vi "2019RefLoopPulseGen.vi"() -> ()   [LabVIEW 2017]
uses:
  offset_parameters.ctl
  Utility Sub VIs/pressure_temp_mixture.ctl
  Utility Sub VIs/pulse_generator_multiheater_controls.ctl
  Utility Sub VIs/pulse_generator_data.ctl
  Utility Sub VIs/pulse_generator_data_charts.ctl
  Utility Sub VIs/pulse_generator_data_controls.ctl
  Input Channel Lists/float_switch_physical_channels.ctl
  Input Channel Lists/pg_control_physical_channels.ctl
  Input Channel Lists/valve_physical_channels.ctl
  Input Channel Lists/window_heater_physical_channels.ctl
  Input Channel Lists/pg_motor_controller_physical_channel.ctl
  Utility Sub VIs/windows_heater_safety_values.ctl
  Utility Sub VIs/window_heaters_control.ctl
  Utility Sub VIs/power_supply_panel.ctl
  Utility Sub VIs/visual_loop.ctl
  Utility Sub VIs/diode_charts.ctl
  Utility Sub VIs/valve_pid_control.ctl
  <vilib>/Utility/error.llb/DialogType.ctl
  Input Channel Lists/label_array_cluster.ctl
  Utility Sub VIs/pulse_generator_controls_multiheater_refnums.ctl
  <vilib>/Utility/sysdir.llb/System Directory Type.ctl
  <vilib>/DAQmx/read.llb/DAQmx Read (Analog 1D Wfm NChan NSamp).vi
  <vilib>/Utility/file.llb/Write Delimited Spreadsheet (string).vi
  <vilib>/DAQmx/configure/timing.llb/DAQmx Timing (Sample Clock).vi
  <vilib>/DAQmx/miscellaneous.llb/DAQmx Fill In Error Info.vi
  <vilib>/NI Modbus.llb/MB Ethernet Master Query Read Holding Registers (poly).vi
  <vilib>/NI Modbus.llb/MB Ethernet Master Query Read Coils (poly).vi
  <vilib>/NI Modbus.llb/MB Ethernet Master Query Write Multiple Registers (poly).vi
  <vilib>/NI Modbus.llb/MB Ethernet Master Query Write Single Coil (poly).vi
  Stop_Global_Variable.vi
  <resource>/objmgr/daqmx.rc
  <vilib>/dex/Stream Element Allocation Mode.ctl
panel:
  in  "Data Saving Parameters":T1={"Sampling\nFrequency"=2000.0, "Recording Duration [s]"=1.0, "Data Index"=1, "Data Prefix"="test", "Data Folder"=path "M:/Annular Flow/Data", "Record Data"=FALSE, "Data Recording Progress"=0, "Notes: "=""} {"Data Recording Progress" scale=0.0..200000.0}
  out "notifier out":refnum<notifier>
  out "Float 5":bool
  out "Float 4":bool=TRUE
  out "Float 3":bool=TRUE
  out "Float 2":bool=TRUE
  out "Float 1":bool=TRUE
  out "Pulse Generator":u8(slide)=80 scale=0.0..100.0 scale format="%.0f%"
  out "Valve Voltage Output":dbl[](array[numeric])=[1.0, 1.0, 1.0]
  out "dataQueue":refnum<queue>
  out "autoOffsetPsatQueue":refnum<queue>
  out "start time":timestamp=timestamp(3643889234.74644 s since 1904-01-01)
  out "Seconds Since\nSession Start":dbl=73.0092568397522
  out "Time Stamp":timestamp=timestamp(3643889307.755697 s since 1904-01-01) format="%<%H:%M:%S%1u>T"
  out "Data Labels":string[][](array[string])=[["", "@(x)(12.000000*(x-0.000000)+0.000000)*6894.757290", "@(y)(y/6894.757290-0.000000)/12.000000+0.000000", "@(x)(626.174076*(x-0.004030)+0.000000)*248.840000", "@(y)(y/248.840000-0.000000)/626.174076+0.004030", "@(x)(1.000000*(x-0.000000)+0.000000)*1.000000", "@(y)(y/1.000000-0.000000)/1.000000+0.000000", "@(x)(1.000000*(x-0.000000)+0.000000)*1.000000", "@(y)(y/1.000000-0.000000)/1.000000+0.000000", "@(x)(1250.000000*(x-0.004000)+0.000000)*248.840000", "@(y)(y/248.840000-0.000000)/1250.000000+0.004000", "@(x)(156.250000*(x-0.004000)+0.000000)*6894.757290", "@(y)(y/6894.757290-0.000000)/156.250000+0.004000", "@(x)(1250.000000*(x-0.004000)+0.000000)*248.840000", "@(y)(y/248.840000-0.000000)/1250.000000+0.004000", "@(x)(1.000000*(x-0.000000)+0.000000)*1.000000", "@(y)(y/1.000000-0.000000)/1.000000+0.000000", "@(x)(1.000000*(x-0.000000)+0.000000)*1.000000", "@(y)(y/1.000000-0.000000)/1.000000+0.000000", "@(x)(10.000000*(x-0.000000)+0.000000)*6894.757290", "@(y)(y/6894.757290-0.000000)/10.000000+0.000000", "@(x)(10.000000*(x-0.000000)+0.000000)*6894.757290", "@(y)(y/6894.757290-0.000000)/10.000000+0.000000", "@(x)(0.200000*(x-0.050000)+0.000000)*6894.757290", "@(y)(y/6894.757290-0.000000)/0.200000+0.050000", "@(x)(5.000000*(x-0.000000)+0.000000)*1.000000", "@(y)(y/1.000000-0.000000)/5.000000+0.000000", "@(x)", "@(y)", "@(x)(1.000000*(x-0.000000)+0.000000)*1.000000", "@(y)(y/1.000000-0.000000)/1.000000+0.000000", "@(x)(1.000000*(x-0.000000)+0.000000)*1.000000", "@(y)(y/1.000000-0.000000)/1.000000+0.000000", "@(x)(1.000000*(x-0.000000)+0.000000)*1.000000", "@(y)(y/1.000000-0.000000)/1.000000+0.000000", "@(x)(1.000000*(x-0.000000)+0.000000)*1.000000", "@(y)(y/1.000000-0.000000)/1.000000+0.000000", "@(x)(23624.581250*(x-0.004000)+0.000000)*1.000000", "@(y)(y/1.000000-0.000000)/23624.581250+0.004000", "@(x)(125.000000*(x-0.004000)+0.000000)*1.000000", "@(y)(y/1.000000-0.000000)/125.000000+0.004000", "@(x)(23624.581250*(x-0.004000)+0.000000)*1.000000", "@(y)(y/1.000000-0.000000)/23624.581250+0.004000", "@(x)(125.000000*(x-0.004000)+0.000000)*1.000000", "@(y)(y/1.000000-0.000000)/125.000000+0.004000", "@(x)(1.000000*(x-0.000000)+0.000000)*1.000000", "@(y)(y/1.000000-0.000000)/1.000000+0.000000", "@(x)(10.000000*(x-0.000000)+0.000000)*6894.757290", "@(y)(y/6894.757290-0.000000)/10.000000+0.000000", "@(x)(1.000000*(x-0.000000)+0.000000)*1.000000", "@(y)(y/1.000000-0.000000)/1.000000+0.000000", "@(x)(10.000000*(x-0.000000)+0.000000)*6894.757290", "@(y)(y/6894.757290-0.000000)/10.000000+0.000000", "@(x)(1.000000*(x-0.000000)+0.000000)*1.000000", "@(y)(y/1.000000-0.000000)/1.000000+0.000000", "@(x)(10.000000*(x-0.000000)+0.000000)*6894.757290", "@(y)(y/6894.757290-0.000000)/10.000000+0.000000", "@(x)(1.000000*(x-0.000000)+0.000000)*1.000000", "@(y)(y/1.000000-0.000000)/1.000000+0.000000", "@(x)(12.000000*(x-0.000000)+0.000000)*6894.757290", "@(y)(y/6894.757290-0.000000)/12.000000+0.000000", "@(x)(10.000000*(x-0.000000)+0.000000)*6894.757290", "@(y)(y/6894.757290-0.000000)/10.000000+0.000000", "@(x)(6.250000*(x-1.000000)+0.000000)*6894.757290", "@(y)(y/6894.757290-0.000000)/6.250000+1.000000", "@(x)", "@(y)", "@(x)(10.000000*(x-0.000000)+0.000000)*6894.757290", "@(y)(y/6894.757290-0.000000)/10.000000+0.000000", "@(x)(1.000000*(x-0.000000)+0.000000)*1.000000", "@(y)(y/1.000000-0.000000)/1.000000+0.000000", "@(x)(10.000000*(x-0.000000)+0.000000)*6894.757290", "@(y)(y/6894.757290-0.000000)/10.000000+0.000000", "@(x)(1.000000*(x-0.000000)+0.000000)*1.000000", "@(y)(y/1.000000-0.000000)/1.000000+0.000000", "@(x)(1.000000*(x-0.000000)+0.000000)*1.000000", "@(y)(y/1.000000-0.000000)/1.000000+0.000000"], ["Timestamp", "PGAbsolutePressure Raw", "PGAbsolutePressure", "VenturidP Raw", "VenturidP", "PGVaporTemperature Raw", "PGVaporTemperature", "PGLiquidTemperature Raw", "PGLiquidTemperature", "Window1to4dP Raw", "Window1to4dP", "Window1to7FastdP Raw", "Window1to7FastdP", "Window1to7dP Raw", "Window1to7dP", "CH4 Raw", "CH4", "CH5 Raw", "CH5", "TSWindow1AbsolutePressure Raw", "TSWindow1AbsolutePressure", "TSWindow7AbsolutePressure Raw", "TSWindow7AbsolutePressure", "DwyerdP Raw", "DwyerdP", "CameraVoltage Raw", "CameraVoltage", "Power Raw", "Power", "MainDiode Raw", "MainDiode", "ControlDiode Raw", "ControlDiode", "TSExteriorTemperature Raw", "TSExteriorTemperature", "DSExteriorTemperature Raw", "DSExteriorTemperature", "VaporMassFlow Raw", "VaporMassFlow", "VaporLineDensity Raw", "VaporLineDensity", "LiquidMassFlow Raw", "LiquidMassFlow", "LiquidLineDensity Raw", "LiquidLineDensity", "MegaTankTemperature Raw", "MegaTankTemperature", "MegaTankPressure Raw", "MegaTankPressure", "SeparatorTemperature Raw", "SeparatorTemperature", "SeparatorPressure Raw", "SeparatorPressure", "LiquidInletTemperature Raw", "LiquidInletTemperature", "LiquidInletPressure Raw", "LiquidInletPressure", "UpperDevSectionTemperature Raw", "UpperDevSectionTemperature", "UpperDevSectionPressure Raw", "UpperDevSectionPressure", "LowerDevSectionPressure Raw", "LowerDevSectionPressure", "AtmosphericPressure Raw", "AtmosphericPressure", "MixingTeedP Raw", "MixingTeedP", "PGinlet-MixingTeePressure Raw", "PGinlet-MixingTeePressure", "PGinlet-MixingTeeTemperature Raw", "PGinlet-MixingTeeTemperature", "TestSectionPressure Raw", "TestSectionPressure", "CH8 Raw", "CH8", "CH9 Raw", "CH9"]]
  in  "Tab Control":T2(tab)=enum."Pulse Generator Data"
  in  "Tabulated/Visualized":enum32{"Tabulated", "Visualized"}(tab)
  in  "Zero Pressure Offsets":bool
  in  "Zero Temp Offsets":bool
  out "Pressure/Temperature/Mixture Properties":T3={"Line Densities\n[g/cm^3]"={"Vapor Line"=-0.500242358953125, "Liquid Line"=-0.5002218156718748}, "Mixture Properties"={"Enthalpy"=328364.73121574003, "Quality [-]"=0.5342547124001654}, "Component PTs"={"Liquid Tank P"=-238.37326971310944, "Liquid Tank T"=19.354366294786907, "Liquid Tank Sat P"=119198.0966686119, "Liquid Tank Sat T"=nan, "Separator P"=641.3597640511042, "Separator T"=19.076846611835087, "Separator Sat P"=117956.20227295622, "Separator Sat T"=-123.53943823013691, "Liquid Inlet P"=-411.8632841584256, "Liquid Inlet T"=19.379355794062125, "Liquid Inlet Sat P"=119310.56377459057, "Liquid Inlet Sat T"=nan, "Vapor Tank P"=-6643.862400161957, "Vapor Tank T"=19.22986162222596, "Vapor Tank Sat P"=118639.33205152737, "Vapor Tank Sat T"=nan, "Vapor Inlet P"=-6643.862400161957, "Vapor Inlet T"=19.22986162222596, "Vapor Inlet Sat P"=118639.33205152737, "Vapor Inlet Sat T"=nan, "Test Section P"=1430.2440274795968, "Test Section T"=0.0, "Test Section Sat P"=57418.5, "Test Section Sat T"=-101.60350769439742, "Upper Dev Section P"=-36.154383120368585, "Upper Dev Section T"=19.182874456914785, "Upper Dev Section Sat P"=118429.13976409887, "Upper Dev Section Sat T"=nan, "Lower Dev Section P"=893.1891396173642, "Lower Dev Section T"=19.182874456914785, "Lower Dev Section Sat P"=118429.13976409887, "Lower Dev Section Sat T"=-114.48050725695731}, "Ambient Pressure [Pa]"=-43212.87918250694, "Mixing Tee"={"Venturi dP"=0.0, "PGminiPressure"=-6216.731665575269, "PGminiTemperature"=19.20694540664635}}
  in  "Auto Offset":bool
  in  "Offset Parameters":T4
  out "Auto Offset Progress":u32(slide) scale=0.0..20.0
  out "# of Datasets Processed":i32=689
  out "Visual Loop Display":T5={"VpTkTemp"=19.22986162222596, "VpTkPres"=-6642.107688688032, "LiqTkTemp"=19.354366294786907, "LiqTkPres"=-236.9015763087729, "PGVapTemp"=18.97439824494449, "PgPres"=-41.11285782633792, "VapInTemp"=19.22986162222596, "VapInPres"=-6642.107688688032, "SepTemp"=19.076846611835087, "SepPres"=645.718240655613, "TSInTemp"=897.2079946562989, "TSInPres"=-34.66004827761057, "LiqInTemp"=19.379355794062125, "LiqInPres"=-398.1086111909236, "DevTemp"=0.0, "DevPres"=0.0, "TSTemp"=0.0, "TSPres"=-43212.631541789204, "Win1-4dP"=-1244.3220538504256, "Win1-7dP"=-1244.2479135883311, "LiqMass"=-94.5155482165204, "VpMass"=-94.52992640457187, "PGMass"=0.0, "PGLiqTemp"=18.479944435977327}
  out "Camera Voltage":dbl[](graph)=[9.625728031, 9.627001843, 9.627638749, 9.629549467, 9.630823279, 9.631778638, 9.631460185, 9.633370903, 9.633689356, 9.633689356, 9.634007809, 9.633370903, 9.633370903, 9.633689356, 9.632415544, 9.632733997, 9.632415544, 9.631778638, 9.630186373, 9.631141732, 9.629231014, 9.628275655, 9.62668339, 9.624772672, 9.62349886, 9.622543501, 9.622225048, 9.622225048, 9.622543501, 9.624135766, 9.625091125, 9.625409578000001, 9.627001843, 9.627638749, 9.629231014, 9.628594108, 9.630186373, 9.631460185, 9.632733997, 9.632733997, 9.633370903, 9.634326262, 9.634007809, 9.634644715, 9.634326262, 9.634963168, 9.635281621, 9.634644715, 9.634007809, 9.633689356, 9.633052450000001, 9.631141732, 9.631141732, 9.629231014, 9.627320296, 9.625728031, 9.624454219, 9.623180407, 9.621906595, 9.620951236, 9.620632783, 9.620951236, 9.622225048, 9.623180407, 9.62349886, 9.624454219, 9.626046484, 9.627638749, 9.628275655, 9.62986792, 9.631141732, 9.632097091, 9.633052450000001, 9.634007809, 9.634326262, 9.634644715, 9.635600074000001, 9.635281621, 9.635600074000001, 9.634963168, 9.634644715, 9.633689356, 9.633689356, 9.633052450000001, 9.632733997, 9.631460185, 9.630504826000001, 9.628912561, 9.627001843, 9.625728031, 9.62349886, 9.621906595, 9.620951236, 9.620632783, 9.620951236, 9.620314330000001, 9.621906595, 9.622861954000001, 9.624135766, 9.624772672, 9.626046484, 9.627957202000001, 9.628912561, 9.630186373, 9.631141732, 9.632097091, 9.632733997, 9.633370903, 9.634963168, 9.635281621, 9.635600074000001, 9.635918527, 9.635600074000001, 9.635918527, 9.635918527, 9.634326262, 9.634326262, 9.632733997, 9.632097091, 9.631141732, 9.62986792, 9.628275655, 9.62668339, 9.624772672, 9.622861954000001, 9.622225048, 9.621588142, 9.621588142, 9.621906595, 9.621588142, 9.622543501, 9.623180407, 9.62349886, 9.625091125, 9.62668339, 9.628594108, 9.628912561, 9.630504826000001, 9.631778638, 9.632097091, 9.633052450000001, 9.633689356, 9.634326262, 9.634644715, 9.634326262, 9.634963168, 9.635281621, 9.634963168, 9.634644715, 9.634644715, 9.634644715, 9.634007809, 9.632415544, 9.630504826000001, 9.629549467, 9.627957202000001, 9.625091125, 9.624135766, 9.622543501, 9.621269689, 9.620951236, 9.621906595, 9.622225048, 9.622543501, 9.62349886, 9.624454219, 9.625409578000001, 9.626364937, 9.627001843, 9.627320296, 9.628912561, 9.630186373, 9.631141732, 9.631778638, 9.632097091, 9.632415544, 9.633052450000001, 9.633689356, 9.634326262, 9.634326262, 9.634326262, 9.634326262, 9.633689356, 9.633052450000001, 9.632415544, 9.631778638, 9.630823279, 9.629549467, 9.628275655, 9.62668339, 9.625409578000001, 9.624135766, 9.622225048, 9.622543501, 9.621906595, 9.622225048, 9.622861954000001, 9.62349886, 9.624135766, 9.625091125]
  out "Vapor Mass Flow Rate":T6(graph)={"Flow Set Point [g/s]"=0.0, "Flow rate [g/s]"=-94.52992640457187}
  out "Liquid Mass Flow Rate":T6(graph)={"Flow Set Point [g/s]"=0.0, "Flow rate [g/s]"=-94.5155482165204}
  in  "Vapor PID Control":T7={"Flow"={"Flow rate [g/s]"=-1.9246389316910921, "Line Density [g/cm^3]"=-0.002869791468750044}, "Valve On/Off"=FALSE, "PID Mode"=FALSE, "PLC Calc Basis"=FALSE, "Flow Set Point [g/s]"=0.0, "Pump Output [%]"=0.0, "Valve Open Voltage [V]"=3.0, "Flow Setpoint Adrs"=28872, "Pump Output Adrs"=28888, "Manual Mode Request Adrs"=16499, "Manual Mode Adrs"=16509} {"Manual Mode Adrs" format="%04x"; "Manual Mode Request Adrs" format="%04x"; "Pump Output Adrs" format="%04x"; "Flow Setpoint Adrs" format="%04x"; "Pump Output [%]" format="%.2f"; "Valve Open Voltage [V]" format="%.2f"; "Flow Set Point [g/s]" format="%.2f"}
  in  "Liquid PID Control":T7={"Flow"={"Flow rate [g/s]"=-1.0242726493384742, "Line Density [g/cm^3]"=-0.004113620409999996}, "Valve On/Off"=FALSE, "PID Mode"=FALSE, "PLC Calc Basis"=FALSE, "Flow Set Point [g/s]"=0.0, "Pump Output [%]"=0.0, "Valve Open Voltage [V]"=3.0, "Flow Setpoint Adrs"=29072, "Pump Output Adrs"=29088, "Manual Mode Request Adrs"=16599, "Manual Mode Adrs"=16609} {"Manual Mode Adrs" format="%04x"; "Manual Mode Request Adrs" format="%04x"; "Pump Output Adrs" format="%04x"; "Flow Setpoint Adrs" format="%04x"; "Pump Output [%]" format="%.2f"; "Valve Open Voltage [V]" format="%.2f"; "Flow Set Point [g/s]" format="%.2f"}
  in  "Pulse Generator Offsets":T8
  out "Measurements Data":T9={"PG Abs Pressure"=-40.9090848933398, "Vapor Temperature"=18.97439824494449, "Liquid Temperature"=18.479944435977327, "PG Supply Temperature"=-40.9090848933398, "Tinlet"=19.436676396501205, "Tsectwo"=19.49953546420568, "TS Abs Pressure W1"=-1394.614861114431, "TS Abs Pressure W7"=-1377.577180233669, "W1-4 dP[Pa]"=-1244.1716334686469, "W1-7 dP[Pa]"=-1244.2994051226024, "W1-7 dP[Pa] Fast"=-4312.785111999902, "PG Venturi dP [Pa]"=-627.9412171524315, "Vapor Line Pitot dP [Pa]"=-161.6047258814074, "Tsecthree"=19.191961040039615, "Toutlet"=19.148186089917207, "TS Ext"=18.97439824494449, "Vapor Sat Pressure"=117501.0252097072, "Liquid Sat Pressure"=115328.74681540662, "PG Mass Flow Rate"=0.0, "Vapor Line Mass Flow"=0.0}
  out "Pulse Generator Charts":T10={"Vapor Mass Flow Rates"={"max value"=0.0, "max value"=0.0}, "Test Section Thermocouples"={"[0]"=19.436676396501205, "[1]"=19.49953546420568, "[2]"=18.939848584535856, "[3]"=19.191961040039615, "[4]"=19.148186089917207}, "Pulse Generator Abs Pressure"=[-40.9090848933398], "Test Section Saturation Pressures"={"max value"=119568.94045291988, "max value"=119852.92544400034}}
  out "Diode Charts":T11={"Liquid Diodes"={10.35690505599997, 10.45756001099999}, "Liquid Intensity Ratio"=0.9903749101229978, "Vapor Diode"={0.0, 0.0}, "Vapor Intensity Ratio"=0.0, "TS Window 1 Temperatures"={"Average"=18.939848584535856, "T Sat [C]"=nan}}
  in  "Commit Settings":bool
  in  "Settings Subpanel":T12(tab)
  in  "Input":T14={"Float Switch Physical Channels"={"Float Line 1"="Input/port0/line0", "Float Line 2"="Input/port0/line1", "Float Line 3"="Input/port0/line2", "Float Line 4"="Input/port0/line3", "Float Line 5"="Input/port0/line4"}, "Float Switch Line Mode"=TRUE}
  in  "Output":T19={"Pulse Generator Control Physical Channels"={"1000W 1"="Output/port0/line1", "1000W 2"="Output/port0/line2", "1000W 3"="Output/port0/line3", "500W 1"="Output/port0/line4", "250W 1"="Output/port0/line5", "150W 1"="Output/port0/line6", "Counter Line"="cDAQ1Mod1/ctr0", "Direction Line"="cDAQ1Mod1/port0/line2"}, "Proportional Valve Physical Channels"={"Vapor Valve"="cDAQ1Mod3/ao1", "Liquid Valve"="cDAQ1Mod3/ao2"}, "Window Heaters Physical Channels"={"Front PS"="COM8", "Rear PS"="COM5"}, "Diode Communication"={"URL"="", "Serial"=""}, "PLC Communication"={"Remote IP"="192.168.0.10", "Remote Port"=502}, "PG Motor Controller Physical Channels"={"USB controller"="COM11"}}
  in  "Safety":T21={"Pulse Generator Heater Safety Values"={"Absolute Pulse Generator Pressure Limit"=250000.0, "Seconds Allowed Pulse Generator Excess Pressure"=60.0, "Absolute Pulse Generator Temperature Limit"=35.0}, "Window Heater Safety Values"={"Minimum Test Section Mass Flow "=1.0, "Maximum Test Section Temperature"=60.0}}
  in  "Import offsets":bool
  in  "Export offsets":bool
  in  "Generate MATLAB Parsing Script":bool
  in  "Open Brians VI":bool
  out "Buffer Overflow":bool
  in  "Run Log":T22(array[cluster])
  out "System Running":bool
  out "error out":errorcluster
  out "Loop Time [ms]":u32=96
  in  "Stop":bool
  in  "Tab Control 2":T23(tab)
  in  "Pulse Generator Controls":T24={"Start Pulse"=FALSE, "Stop Pulse"=FALSE, "Pulse Gen\nActive?"=FALSE, "Steady Frequency [Hz]"=10.0, "Ramp Duration [s]"=5.0, "Steady Duration[s]"=10.0, " Motor Dir"=FALSE, "Heaters"=FALSE, "Heater ON?"=FALSE, "1000-1"=FALSE, "1000-2"=FALSE, "1000-3"=FALSE, "500-1"=FALSE, "250-1"=FALSE, "150-1"=FALSE, "Hysteresis"=10.0, "PG Controller Switch"=FALSE, "Power [W]"=0.0, "Start Frequency [Hz]"=1.0, "Pulse Mode"=FALSE, "Frequency [Hz]"=0.0, "+/- % Movement"=90.0, "Repetitions"=20, "Average % Open"=90.0, "1000W 1 PID"=FALSE, "1000W 2 PID"=FALSE, "1000W 3 PID"=FALSE, "500W 1 PID"=FALSE, "250W 1 PID"=FALSE, "150W 1 PID"=FALSE, "Setpoint [Pa]"=130000.0} {"Setpoint [Pa]" min=1.0 max=5.0; "Average % Open" min=1.0 step=500.0; "+/- % Movement" min=1.0 step=500.0; "Start Frequency [Hz]" min=1.0 step=500.0; "Power [W]" min=1.0 max=5.0 format="%.2f"; "Hysteresis" min=0.0 max=5.0; "Steady Frequency [Hz]" min=1.0 step=500.0}
  in  "Window Heaters Control":T25={"Window Heater Switch"=FALSE, "Safety Trigger"=FALSE, "Front Readout"={"Voltage High Limit"=10.0, "Current High Limit"=10.0, "Power Setpoint"=2.0, "Voltage"=10.005, "Current"=0.0, "Power"=0.0}, "Rear Readout"={"Voltage High Limit"=10.0, "Current High Limit"=10.0, "Power Setpoint"=2.0, "Voltage"=9.99, "Current"=0.0007, "Power"=0.0}, "Reset PS Error"=FALSE}
  in  "Offsets":T27(array[cluster])=[{"Channel"="VaporMassFlow", "Offset"=0.0, "Output Unit"=enum."g/s"}, {"Channel"="VaporLineDensity", "Offset"=0.0, "Output Unit"=enum."g/cm3"}, {"Channel"="LiquidMassFlow", "Offset"=0.0, "Output Unit"=enum."g/s"}, {"Channel"="LiquidLineDensity", "Offset"=0.0, "Output Unit"=enum."g/cm3"}, {"Channel"="VaporInletPressure", "Offset"=0.0, "Output Unit"=enum."Pa"}, {"Channel"="MegaTankPressure", "Offset"=0.0, "Output Unit"=enum."Pa"}, {"Channel"="SeparatorPressure", "Offset"=0.0, "Output Unit"=enum."Pa"}, {"Channel"="LiquidInletPressure", "Offset"=0.0, "Output Unit"=enum."Pa"}, {"Channel"="VaporInletTemperature", "Offset"=0.0, "Output Unit"=enum."C"}, {"Channel"="MegaTankTemperature", "Offset"=0.0, "Output Unit"=enum."C"}, {"Channel"="LiquidInletTemperature", "Offset"=0.0, "Output Unit"=enum."C"}, {"Channel"="SeparatorTemperature", "Offset"=0.0, "Output Unit"=enum."C"}, {"Channel"="LowerDevSectionPressure", "Offset"=0.0, "Output Unit"=enum."Pa"}, {"Channel"="UpperDevSectionTemperature", "Offset"=0.0, "Output Unit"=enum."C"}, {"Channel"="UpperDevSectionPressure", "Offset"=0.0, "Output Unit"=enum."Pa"}, {"Channel"="TestSectionTemperature", "Offset"=0.0, "Output Unit"=enum."C"}, {"Channel"="TestSectionPressure", "Offset"=0.0, "Output Unit"=enum."Pa"}, {"Channel"="DwyerdP", "Offset"=0.0, "Output Unit"=enum."Pa"}, {"Channel"="VenturidP", "Offset"=0.0, "Output Unit"=enum."Pa"}, {"Channel"="PGinlet-MixingTeePressure", "Offset"=0.0, "Output Unit"=enum."Pa"}, {"Channel"="PGinlet-MixingTeeTemperature", "Offset"=0.0, "Output Unit"=enum."C"}, {"Channel"="AtmosphericPressure", "Offset"=0.0, "Output Unit"=enum."Pa"}, {"Channel"="PGAbsolutePressure", "Offset"=0.0, "Output Unit"=enum."Pa"}, {"Channel"="PGVaporTemperature", "Offset"=0.0, "Output Unit"=enum."C"}, {"Channel"="PGLiquidTemperature", "Offset"=0.0, "Output Unit"=enum."C"}, {"Channel"="Window1to4dP", "Offset"=0.0, "Output Unit"=enum."Pa"}, {"Channel"="Window1to7dP", "Offset"=0.0, "Output Unit"=enum."Pa"}, {"Channel"="Window1to7FastdP", "Offset"=0.0, "Output Unit"=enum."Pa"}, {"Channel"="CameraVoltage", "Offset"=0.0, "Output Unit"=enum."Volt"}, {"Channel"="CH4", "Offset"=0.0, "Output Unit"=enum."C"}, {"Channel"="CH5", "Offset"=0.0, "Output Unit"=enum."C"}, {"Channel"="TSWindow1AbsolutePressure", "Offset"=0.0, "Output Unit"=enum."Pa"}, {"Channel"="TSWindow7AbsolutePressure", "Offset"=0.0, "Output Unit"=enum."Pa"}, {"Channel"="MainDiode", "Offset"=0.0, "Output Unit"=enum."Volt"}, {"Channel"="ControlDiode", "Offset"=0.0, "Output Unit"=enum."Volt"}, {"Channel"="TSExteriorTemperature", "Offset"=0.0, "Output Unit"=enum."C"}, {"Channel"="DSExteriorTemperature", "Offset"=0.0, "Output Unit"=enum."C"}, {"Channel"="PostMixingTeeTemperature", "Offset"=0.0, "Output Unit"=enum."Volt"}, {"Channel"="CH8", "Offset"=0.0, "Output Unit"=enum."C"}, {"Channel"="CH9", "Offset"=0.0, "Output Unit"=enum."C"}]
  # "Saturation\nPressure [Pa]"
  # "Saturation\nTemperature [C]"
  # "Pressure [Pa]"
  # "Temperature [C]"
  # "Mega Tank"
  # "Separator"
  # "Liquid Inlet"
  # "Vapor Inlet"
  # "Vapor Inlet"
  # "Test Section"
  # "Upper Dev Section"
  # "Lower Dev Section"
  # "Test Section"
  # "Pulse Gen"
  # "Normal: NC\nInvert: NO\nSwitch 0 is inverted"
  # "NI-9401 Counter & DIO (pin) Chart"
  # "Default Pins used by Counter:\n     SRC: P-Gen Counter Timebase, A-input  \n     GATE: P-Gen Trigger, Z-input\n     AUX: B-input \n     OUT: P_Gen Output\nMore info:  Programs»National Instruments»NI-DAQ»NI-DAQmx Key Concepts»Counters"
  # "0"
  # "1"
  # "2"
  # "3"
  # "7 (25)"
  # "6 (23)"
  # "4 (20)"
  # "5 (22)"
  # "3 (19)"
  # "2 (17)"
  # "0 (14)"
  # "1 (16)"
  # "4 (20)"
  # "5 (22)"
  # "6 (23)"
  # "7 (25)"
  # "0 (14)"
  # "1 (16)"
  # "2 (17)"
  # "3 (19)"
  # "COUNTER"
  # "SRC"
  # "GATE"
  # "AUX"
  # "OUT"
  # "Heater Switches"
  # "Heater P Control"
  # "Current Est Power"
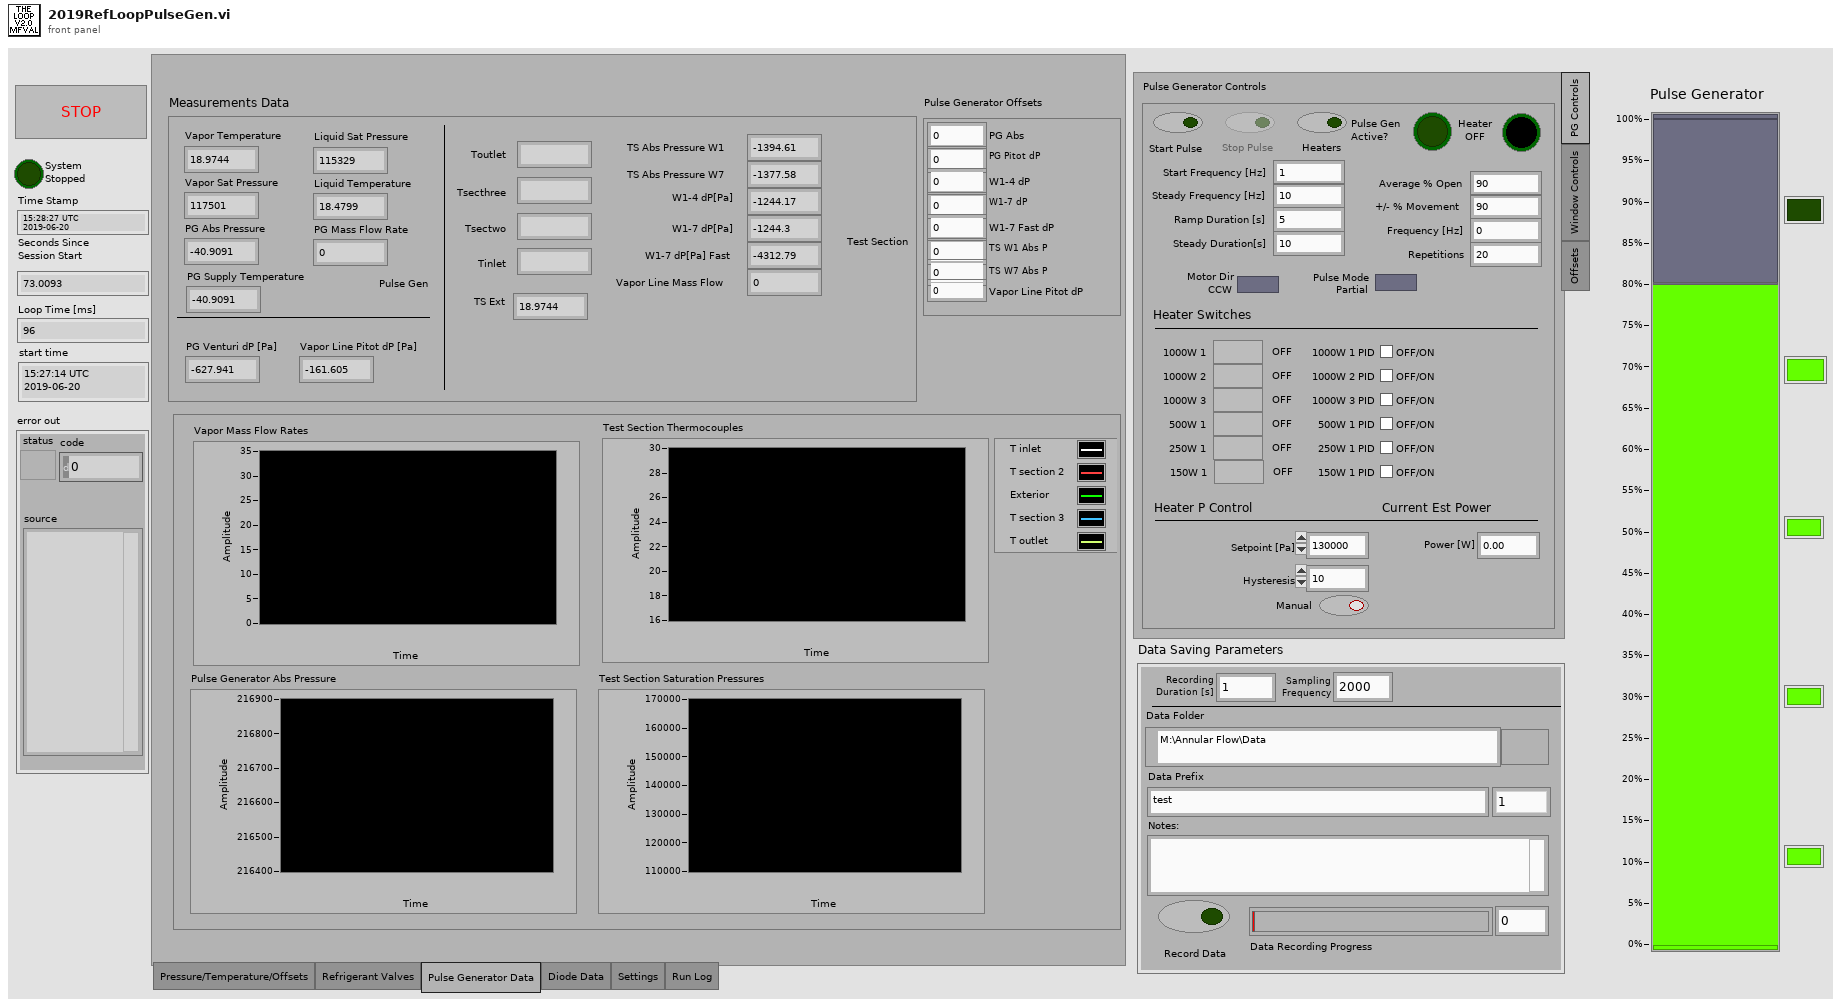
[diagram p1: front panel]
types:
  T1 = cluster{"Sampling\nFrequency":dbl, "Recording Duration [s]":dbl, "Data Index":i32, "Data Prefix":string, "Data Folder":path, "Record Data":bool, "Data Recording Progress":u32, "Notes: ":string}
  T2 = enum32{"Pressure/Temperature/Offsets", "Refrigerant Valves", "Pulse Generator Data", "Diode Data", "Settings", "Run Log"}
  T3 = typedef "pressure_temp_mixture.ctl" = cluster{"Line Densities\n[g/cm^3]":cluster{"Vapor Line":dbl, "Liquid Line":dbl}, "Mixture Properties":cluster{"Enthalpy":dbl, "Quality [-]":dbl}, "Component PTs":cluster{"Liquid Tank P":dbl, "Liquid Tank T":dbl, "Liquid Tank Sat P":dbl, "Liquid Tank Sat T":dbl, "Separator P":dbl, "Separator T":dbl, "Separator Sat P":dbl, "Separator Sat T":dbl, "Liquid Inlet P":dbl, "Liquid Inlet T":dbl, "Liquid Inlet Sat P":dbl, "Liquid Inlet Sat T":dbl, "Vapor Tank P":dbl, "Vapor Tank T":dbl, "Vapor Tank Sat P":dbl, "Vapor Tank Sat T":dbl, "Vapor Inlet P":dbl, "Vapor Inlet T":dbl, "Vapor Inlet Sat P":dbl, "Vapor Inlet Sat T":dbl, "Test Section P":dbl, "Test Section T":dbl, "Test Section Sat P":dbl, "Test Section Sat T":dbl, "Upper Dev Section P":dbl, "Upper Dev Section T":dbl, "Upper Dev Section Sat P":dbl, "Upper Dev Section Sat T":dbl, "Lower Dev Section P":dbl, "Lower Dev Section T":dbl, "Lower Dev Section Sat P":dbl, "Lower Dev Section Sat T":dbl}, "Ambient Pressure [Pa]":dbl, "Mixing Tee":cluster{"Venturi dP":dbl, "PGminiPressure":dbl, "PGminiTemperature":dbl}}
  T4 = typedef "offset_parameters.ctl" = cluster{"Mega Tank\nPressure":dbl, "Mega Tank\nTemperature":dbl, "Separator Pressure":dbl, "Separator \nTemperature":dbl, "Liquid Inlet\nPressure":dbl, "Liquid Inlet\nTemperature ":dbl, "Vapor Inlet\nPressure ":dbl, "Vapor Inlet\nTemperature ":dbl, "Vapor Inlet\nPressure":dbl, "Vapor Inlet \nTemperature":dbl, "Test Section\nPressure":dbl, "Test Section\nTemperature":dbl, "Upper Dev Section\nPressure":dbl, "Upper Dev Section\nTemperature":dbl, "Lower Dev Section\nPressure":dbl, "PG Inlet-Mixing Tee Pressure":dbl, "Vapor Line dP":dbl, "Atmospheric Pressure [Pa]":dbl}
  T5 = typedef "visual_loop.ctl" = cluster{"VpTkTemp":dbl, "VpTkPres":dbl, "LiqTkTemp":dbl, "LiqTkPres":dbl, "PGVapTemp":dbl, "PgPres":dbl, "VapInTemp":dbl, "VapInPres":dbl, "SepTemp":dbl, "SepPres":dbl, "TSInTemp":dbl, "TSInPres":dbl, "LiqInTemp":dbl, "LiqInPres":dbl, "DevTemp":dbl, "DevPres":dbl, "TSTemp":dbl, "TSPres":dbl, "Win1-4dP":dbl, "Win1-7dP":dbl, "LiqMass":dbl, "VpMass":dbl, "PGMass":dbl, "PGLiqTemp":dbl}
  T6 = cluster{"Flow Set Point [g/s]":dbl, "Flow rate [g/s]":dbl}
  T7 = typedef "valve_pid_control.ctl" = cluster{"Flow":cluster{"Flow rate [g/s]":dbl, "Line Density [g/cm^3]":dbl}, "Valve On/Off":bool, "PID Mode":bool, "PLC Calc Basis":bool, "Flow Set Point [g/s]":dbl, "Pump Output [%]":dbl, "Valve Open Voltage [V]":dbl, "Flow Setpoint Adrs":u16, "Pump Output Adrs":u16, "Manual Mode Request Adrs":u16, "Manual Mode Adrs":u16}
  T8 = typedef "pulse_generator_data_controls.ctl" = cluster{"PG Abs":dbl, "PG Pitot dP":dbl, "W1-4 dP ":dbl, "W1-7 dP":dbl, "W1-7 Fast dP":dbl, "TS W1 Abs P":dbl, "TS W7 Abs P":dbl, "Vapor Line Pitot dP":dbl}
  T9 = typedef "pulse_generator_data.ctl" = cluster{"PG Abs Pressure":dbl, "Vapor Temperature":dbl, "Liquid Temperature":dbl, "PG Supply Temperature":dbl, "Tinlet":dbl, "Tsectwo":dbl, "TS Abs Pressure W1":dbl, "TS Abs Pressure W7":dbl, "W1-4 dP[Pa]":dbl, "W1-7 dP[Pa]":dbl, "W1-7 dP[Pa] Fast":dbl, "PG Venturi dP [Pa]":dbl, "Vapor Line Pitot dP [Pa]":dbl, "Tsecthree":dbl, "Toutlet":dbl, "TS Ext":dbl, "Vapor Sat Pressure":dbl, "Liquid Sat Pressure":dbl, "PG Mass Flow Rate":dbl, "Vapor Line Mass Flow":dbl}
  T10 = typedef "pulse_generator_data_charts.ctl" = cluster{"Vapor Mass Flow Rates":cluster{"max value":dbl, "max value":dbl}, "Test Section Thermocouples":cluster{"[0]":dbl, "[1]":dbl, "[2]":dbl, "[3]":dbl, "[4]":dbl}, "Pulse Generator Abs Pressure":dbl[], "Test Section Saturation Pressures":cluster{"max value":dbl, "max value":dbl}}
  T11 = typedef "diode_charts.ctl" = cluster{"Liquid Diodes":cluster{dbl, dbl}, "Liquid Intensity Ratio":dbl, "Vapor Diode":cluster{dbl, dbl}, "Vapor Intensity Ratio":dbl, "TS Window 1 Temperatures":cluster{"Average":dbl, "T Sat [C]":dbl}}
  T12 = enum32{"Input", "Output", "Safety", "Other Functions"}
  T13 = typedef "float_switch_physical_channels.ctl" = cluster{"Float Line 1":tag, "Float Line 2":tag, "Float Line 3":tag, "Float Line 4":tag, "Float Line 5":tag}
  T14 = cluster{"Float Switch Physical Channels":T13, "Float Switch Line Mode":bool}
  T15 = typedef "pg_control_physical_channels.ctl" = cluster{"1000W 1":tag, "1000W 2":tag, "1000W 3":tag, "500W 1":tag, "250W 1":tag, "150W 1":tag, "Counter Line":tag, "Direction Line":tag}
  T16 = typedef "valve_physical_channels.ctl" = cluster{"Vapor Valve":tag, "Liquid Valve":tag}
  T17 = typedef "window_heater_physical_channels.ctl" = cluster{"Front PS":refnum<visa-resource-name>, "Rear PS":refnum<visa-resource-name>}
  T18 = typedef "pg_motor_controller_physical_channel.ctl" = cluster{"USB controller":refnum<visa-resource-name>}
  T19 = cluster{"Pulse Generator Control Physical Channels":T15, "Proportional Valve Physical Channels":T16, "Window Heaters Physical Channels":T17, "Diode Communication":cluster{"URL":string, "Serial":refnum<visa-resource-name>}, "PLC Communication":cluster{"Remote IP":string, "Remote Port":u16}, "PG Motor Controller Physical Channels":T18}
  T20 = typedef "windows_heater_safety_values.ctl" = cluster{"Minimum Test Section Mass Flow ":dbl, "Maximum Test Section Temperature":dbl}
  T21 = cluster{"Pulse Generator Heater Safety Values":cluster{"Absolute Pulse Generator Pressure Limit":dbl, "Seconds Allowed Pulse Generator Excess Pressure":dbl, "Absolute Pulse Generator Temperature Limit":dbl}, "Window Heater Safety Values":T20}
  T22 = cluster{"File Number":string, "Entry Content":string}[]
  T23 = enum32{"PG Controls", "Window Controls", "Offsets"}
  T24 = typedef "pulse_generator_multiheater_controls.ctl" = cluster{"Start Pulse":bool, "Stop Pulse":bool, "Pulse Gen\nActive?":bool, "Steady Frequency [Hz]":dbl, "Ramp Duration [s]":dbl, "Steady Duration[s]":dbl, " Motor Dir":bool, "Heaters":bool, "Heater ON?":bool, "1000-1":bool, "1000-2":bool, "1000-3":bool, "500-1":bool, "250-1":bool, "150-1":bool, "Hysteresis":dbl, "PG Controller Switch":bool, "Power [W]":dbl, "Start Frequency [Hz]":dbl, "Pulse Mode":bool, "Frequency [Hz]":dbl, "+/- % Movement":dbl, "Repetitions":u32, "Average % Open":dbl, "1000W 1 PID":bool, "1000W 2 PID":bool, "1000W 3 PID":bool, "500W 1 PID":bool, "250W 1 PID":bool, "150W 1 PID":bool, "Setpoint [Pa]":dbl}
  T25 = typedef "window_heaters_control.ctl" = cluster{"Window Heater Switch":bool, "Safety Trigger":bool, "Front Readout":T26, "Rear Readout":T26, "Reset PS Error":bool}
  T26 = typedef "power_supply_panel.ctl" = cluster{"Voltage High Limit":dbl, "Current High Limit":dbl, "Power Setpoint":dbl, "Voltage":dbl, "Current":dbl, "Power":dbl}
  T27 = cluster{"Channel":string, "Offset":dbl, "Output Unit":enum16{"psi", "Pa", "inH2O", "inHg", "C", "K", "g/s", "g/cm3", "Volt", "Amp", ""}}[]
  T28 = enum32{"Pressure/Temperature/Offsets", "Refrigerant Valves", "Pulse Generator Data", "Diode Data", "Settings"}
  T29 = enum8{"Enabled", "Disabled", "Disabled and Grayed Out"}
  T30 = cluster{"max value":dbl, "max value":dbl, "max value":dbl, "max value 2":dbl, "max value 3":dbl}[]
  T31 = enum32{"Pressure/Temperature/Offsets", "Refrigerant Valves", "Pulse Generator Data", "Settings"}
  T32 = cluster{"Channel Name":string, "Label":string, "Offset":dbl, "Raw":dbl[], "Processed":dbl[], "Converted":dbl[], "Average":dbl}
  T33 = typedef "label_array_cluster.ctl" = cluster{"Label Array":string[]}
  T34 = enum32{"Invalid", "Standard", "Closed", "Hidden", "Minimized", "Maximized"}
  T35 = cluster{"Entry Content":string, "File Number":string}
  T36 = typedef "DialogType.ctl" = u16
  T37 = cluster{"Flow Set Point [g/s]":dbl, "Flow rate [g/s]":dbl}[]
  T38 = typedef "analog_data_channel_pkg.ctl" = cluster{"Analog Input Channel":T39, "Analog Data":T40}
  T39 = typedef "input_channel.ctl" = cluster{"Channel Name":string, "Physical Channel":tag, "Sensor Type":enum16{"Absolute Pressure", "Gauge Pressure", "Differential Pressure", "Temperature", "Mass Flow Rate", "Density", "Other"}, "Signal Type":enum16{"Voltage", "Current", "Temperature"}, "Terminal Configuration":i32, "Minimum Value":dbl, "Maximum Value":dbl, "TC Type":i32, "Sensor Min":dbl, "Sensor Max":dbl, "Sensor Offset":dbl, "Sensor Unit":enum16{"psi", "Pa", "inH2O", "inHg", "C", "K", "g/s", "g/cm3", "Volt", "Amp", ""}, "Output Unit":enum16{"psi", "Pa", "inH2O", "inHg", "C", "K", "g/s", "g/cm3", "Volt", "Amp", ""}, "Unit Conversion":dbl, "Active":bool, "Input Type":enum16{"DAQ", "Add-On"}}
  T40 = typedef "analog_data.ctl" = cluster{"Label":string, "Offset":dbl, "Raw":dbl[], "Converted":dbl[], "Average":dbl, "Formula To Output":string, "Formula From Output":string}
  T41 = enum16{"psi", "Pa", "inH2O", "inHg", "C", "K", "g/s", "g/cm3", "Volt", "Amp", ""}
  T42 = cluster{"Label":string, "Offset":dbl, "Output Unit":enum16{"psi", "Pa", "inH2O", "inHg", "C", "K", "g/s", "g/cm3", "Volt", "Amp", ""}}
  T43 = typedef "index_array_cluster.ctl" = cluster{"Index Array":i32[]}
  T44 = typedef "Stream Element Allocation Mode.ctl" = u32
  T45 = cluster{"Flow":cluster{"Flow rate [g/s]":dbl, "Line Density [g/cm^3]":dbl}, "Valve On/Off":bool, "PID Mode":bool, "PLC Calc Basis":bool, "Flow Set Point [g/s]":dbl, "Pump Output [%]":dbl, "Valve Open Voltage [V]":dbl, "Flow Setpoint Adrs":u16, "Pump Output Adrs":u16, "Manual Mode Request Adrs":u16, "Manual Mode Adrs":u16}
  T46 = cluster{"Channel":string, "Offset":dbl, "Output Unit":enum16{"psi", "Pa", "inH2O", "inHg", "C", "K", "g/s", "g/cm3", "Volt", "Amp", ""}}
  T47 = typedef "pulse_generator_controls_multiheater_refnums.ctl" = cluster{"Start Pulse":refnum<vi>, "Stop Pulse":refnum<vi>, "Heaters":refnum<vi>, "Counter":refnum<vi>, "Start Frequency (Hz)":refnum<vi>, "Pulse Generator Active":refnum<vi>, "Stepper Motor Direction":refnum<vi>, "Ramp Duration":refnum<vi>, "Direction Line":refnum<vi>, "1000-1 Line":refnum<vi>, "1000-2 Line":refnum<vi>, "1000-3 Line":refnum<vi>, "500-1 Line":refnum<vi>, "250-1 Line":refnum<vi>, "1000-1":refnum<vi>, "1000-2":refnum<vi>, "1000-3":refnum<vi>, "500-1":refnum<vi>, "250-1":refnum<vi>, "150-1":refnum<vi>, "Heater ON?":refnum<vi>, "150-1 Line":refnum<vi>, "Power":refnum<vi>, "Steady Frequency (Hz)":refnum<vi>, "Steady Duration ":refnum<vi>, "Pulse Mode":refnum<vi>, "Frequency [Hz]":refnum<vi>, "Avg % Open":refnum<vi>, "Repetitions":refnum<vi>, "+/- % Open":refnum<vi>, "USB Controller":refnum<vi>}
  T48 = cluster{"Liquid Tank P":dbl, "Liquid Tank T":dbl, "Liquid Tank Sat P":dbl, "Liquid Tank Sat T":dbl, "Separator P":dbl, "Separator T":dbl, "Separator Sat P":dbl, "Separator Sat T":dbl, "Liquid Inlet P":dbl, "Liquid Inlet T":dbl, "Liquid Inlet Sat P":dbl, "Liquid Inlet Sat T":dbl, "Vapor Tank P":dbl, "Vapor Tank T":dbl, "Vapor Tank Sat P":dbl, "Vapor Tank Sat T":dbl, "Vapor Inlet P":dbl, "Vapor Inlet T":dbl, "Vapor Inlet Sat P":dbl, "Vapor Inlet Sat T":dbl, "Test Section P":dbl, "Test Section T":dbl, "Test Section Sat P":dbl, "Test Section Sat T":dbl, "Upper Dev Section P":dbl, "Upper Dev Section T":dbl, "Upper Dev Section Sat P":dbl, "Upper Dev Section Sat T":dbl, "Lower Dev Section P":dbl, "Lower Dev Section T":dbl, "Lower Dev Section Sat P":dbl, "Lower Dev Section Sat T":dbl}
  T49 = typedef "System Directory Type.ctl" = i32
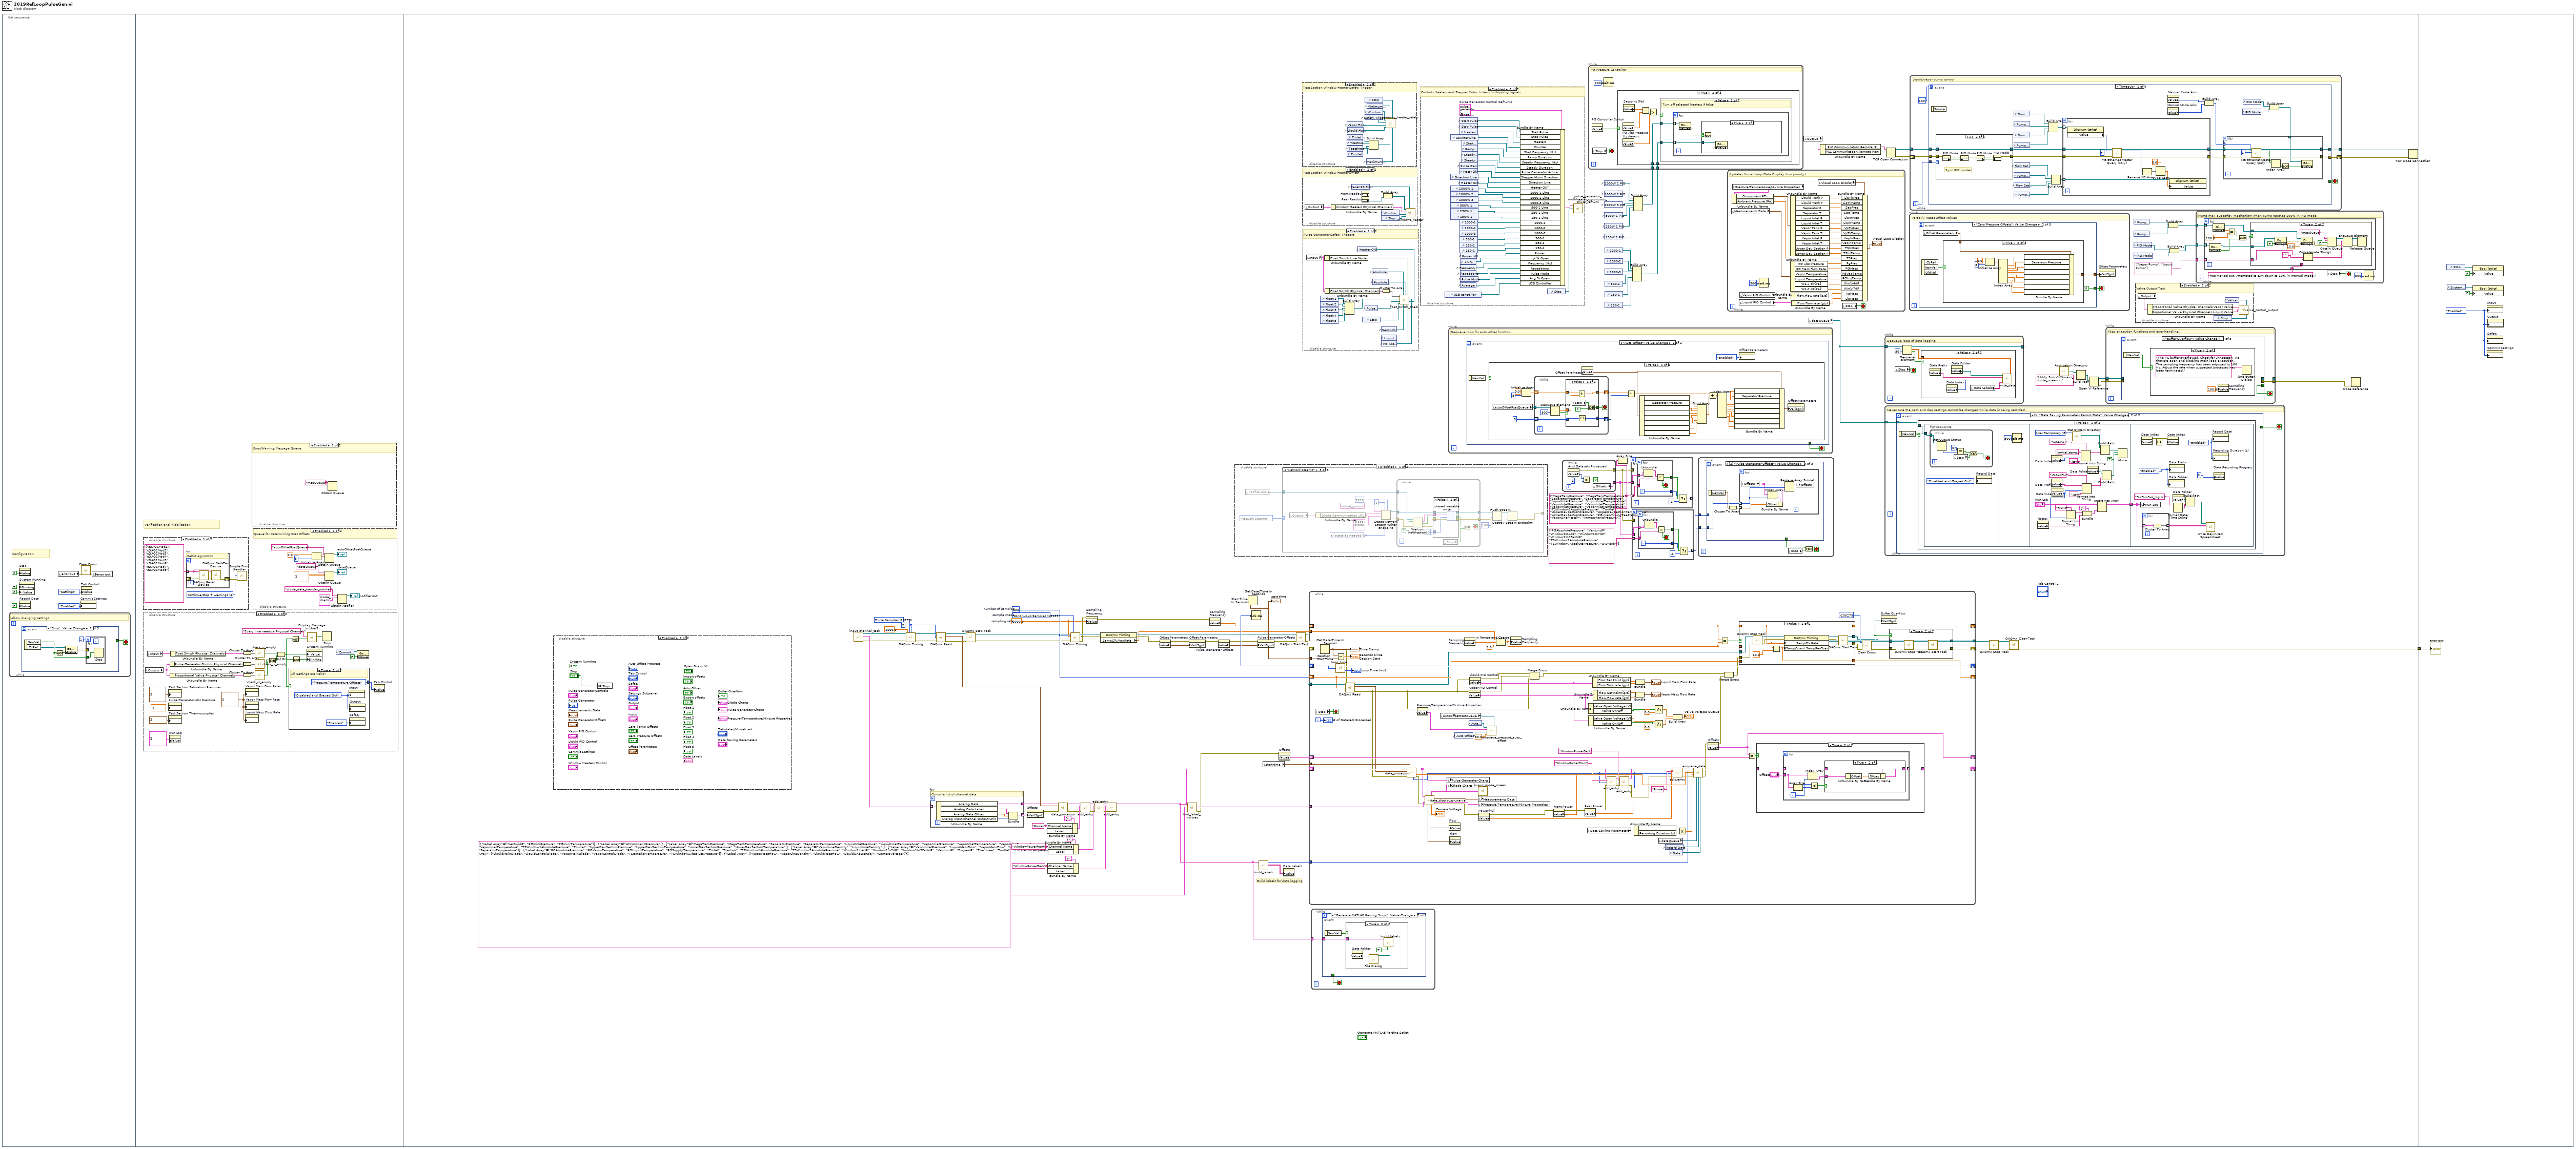
[diagram p0: block diagram]
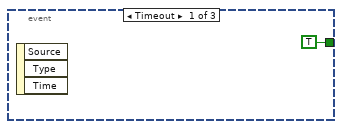
[diagram p2: hidden frame]
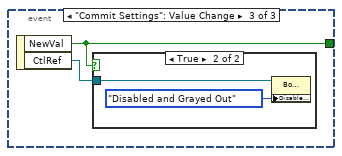
[diagram p3: hidden frame]
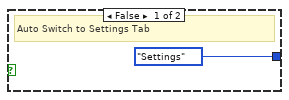
[diagram p7: hidden frame]
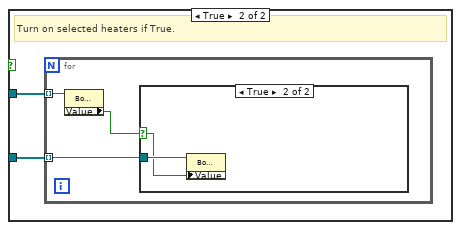
[diagram p13: hidden frame]
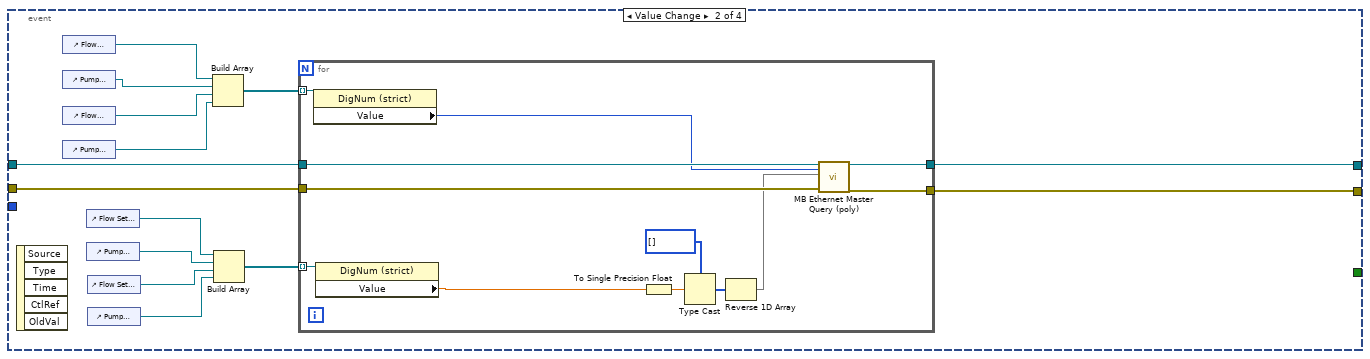
[diagram p16: hidden frame]
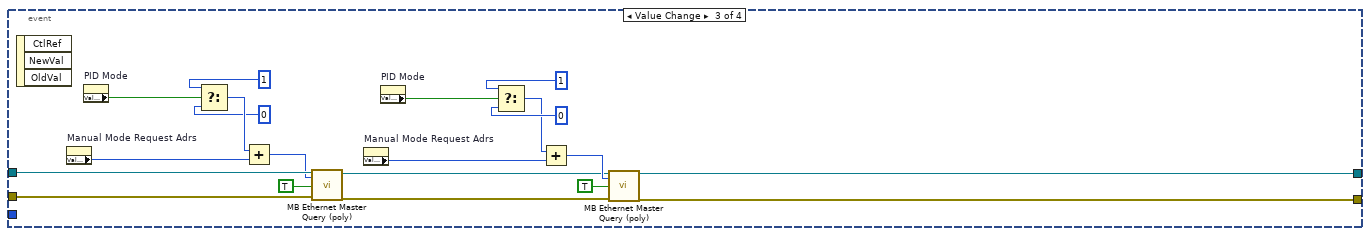
[diagram p17: hidden frame]
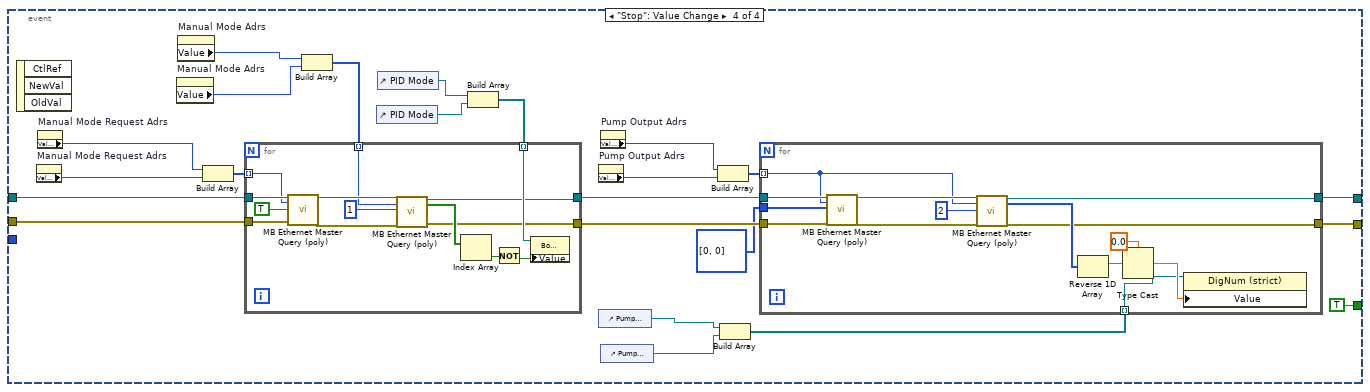
[diagram p18: hidden frame]
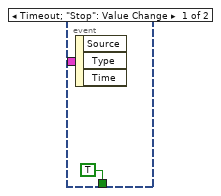
[diagram p19: hidden frame]
diagram:
  n1 = flat-sequence {
    tunnel: [w176] -> w1
    tunnel: w1 -> [w962]
    frame #0 {
      # "Configuration"
      n2 = while {
        stop <- w10 stop-if-true
        # "Allow changing settings"
        n3 = event shown="[1] \"Stop\": Value Change" {
          selector: _ -> [_ _ _]
          dyn-events: _ -> [_ _ _]
          timeout: _ -> [_ _ _]
          tunnel: [TRUE ("NewVal") _ w18] -> w10
          event Timeout {
            n4 = event-data() -> ()  [unwired: 1 in, 3 out]
          }
          event "Stop": Value Change {
            n5 = event-data() -> ("NewVal"=w16:bool, "CtlRef"=w15:refnum<vi>)  [unwired: 1 in]
            n6 = Not(x=w16) -> (.not. x?=w14:bool)
            n7 = property class="Bool (strict)"(reference=w15, "Value"=w14) -> (error out=w13:errorcluster)  [unwired: 1 in, 1 out]
            n8 = for {
              N: 1 -> [_]
              tunnel: w16 -> [w17]
              tunnel: w13 -> [_]
              n9 = Stop(stop? (T)=w17) -> ()
            }
          }
          event "Commit Settings": Value Change {
            n10 = event-data() -> ("NewVal"=w18:bool, "CtlRef"=w19:refnum<vi>)  [unwired: 1 in]
            n11 = case shown="True" w18 {
              tunnel: w19 -> [_ w21]
              frame False {
              }
              frame True {
                n12 = property class="Bool (strict)"(reference=w21, "DisabledEnum"=T29."Disabled and Grayed Out" ("Disabled")) -> ()  [unwired: 1 in, 2 out]
              }
            }
          }
        }
      }
      n13 = property on="Stop" class="Bool (strict)"("Value"=FALSE) -> ()  [unwired: 2 in, 2 out]
      n14 = property on="System Running" class="Bool (strict)"("Blinking"=TRUE ("Value"), "Value"=FALSE) -> ()  [unwired: 2 in, 2 out]
      n15 = property on="Record Data" class="Bool (strict)"("Value"=FALSE) -> ()  [unwired: 2 in, 2 out]
      n16 = local read "error out"() -> (w9:errorcluster)
      n17 = property on="Commit Settings" class="Bool (strict)"("DisabledEnum"=T29."Enabled" ("Disabled")) -> ()  [unwired: 2 in, 2 out]
      n18 = call <vilib>:"Clear Errors.vi"("error in (no error)"=w9) -> ("error out"=w8:errorcluster)  [unwired: 5 in, 1 out]
      n19 = property on="Tab Control" class="TabCtl (strict)"("Value"=T28."Settings" ("Tab Control")) -> ()  [unwired: 2 in, 2 out]
      n20 = local write "error out"(w8) -> ()
    }
    frame #1 {
      # "Verification and initialization"
      n21 = disable-structure shown="Enabled" {
        frame Enabled {
          w63 = T36 4 items=["no dialog", "OK message", "continue or stop message", "OK message + warnings", "continue/stop + warnings"] ("type of dialog (OK msg:1)")
          n22 = for {
            tunnel: string[] ["cDAQ1Mod1", "cDAQ1Mod2", "cDAQ1Mod3", "cDAQ1Mod4", "cDAQ1Mod5", "cDAQ1Mod6", "cDAQ1Mod7", "cDAQ1Mod8"] -> [w67] mode=indexing
            shift-right: [w69] -> w64
            shift-left: _ -> [w66]
            # "Self-Diagnostics"
            n23 = call <vilib>:"DAQmx Reset Device.vi"("device in"=w67, "error in"=w66) -> ("error out"=w68:errorcluster)  [unwired: 13 in]
            n24 = call <vilib>:"DAQmx Self-Test Device.vi"("device in"=w67, "error in"=w68) -> ("error out"=w69:errorcluster)  [unwired: 13 in]
          }
          n25 = call <vilib>:"Simple Error Handler.vi"("type of dialog (OK msg:1)"=w63, "error in (no error)"=w64) -> ()  [unwired: 3 in, 5 out]
        }
        frame Disabled {
        }
      }
      n26 = disable-structure shown="Enabled" {
        frame Enabled {
          w38 = T37 [] ("History Data")
          n27 = local read "Output"() -> (w42:T19)
          n28 = local read "Input"() -> (w47:T14)
          n29 = property on="Test Section Saturation Pressures" class="WFChart (strict)"("History Data"=cluster{"max value":dbl, "max value":dbl}[] []) -> ()  [unwired: 2 in, 2 out]
          n30 = property on="Pulse Generator Abs Pressure" class="WFChart (strict)"("History Data"=dbl[] []) -> ()  [unwired: 2 in, 2 out]
          n31 = property on="Test Section Thermocouples" class="WFChart (strict)"("History Data"=T30 []) -> ()  [unwired: 2 in, 2 out]
          n32 = property on="Run Log" class="Arr (strict)"("Value"=T22 [] ("Run Log")) -> ()  [unwired: 2 in, 2 out]
          n33 = Unbundle By Name(w42) -> ("Pulse Generator Control Physical Channels"=w48:T15)
          n34 = Unbundle By Name(w42) -> ("Proportional Valve Physical Channels"=w46:T16)
          n35 = Unbundle By Name(w47) -> ("Float Switch Physical Channels"=w49:T13)
          n36 = Cluster To Array(cluster=w49) -> (array=w58:tag[])
          n37 = Cluster To Array(cluster=w48) -> (array=w57:tag[])
          n38 = Cluster To Array(cluster=w46) -> (array=w56:tag[])
          n39 = property on="Vapor Mass Flow Rates" class="WFChart (strict)"("History Data"=w38) -> ()  [unwired: 2 in, 2 out]
          n40 = property on="Vapor Mass Flow Rate" class="WFChart (strict)"("History Data"=w38) -> ()  [unwired: 2 in, 2 out]
          n41 = property on="Liquid Mass Flow Rate" class="WFChart (strict)"("History Data"=w38) -> ()  [unwired: 2 in, 2 out]
          n42 = call "check_is_empty.vi"("Channels"=w58) -> ("Has Empty?"=w36:bool)
          n43 = call "check_is_empty.vi"("Channels"=w57) -> ("Has Empty?"=w55:bool)
          n44 = call "check_is_empty.vi"("Channels"=w56) -> ("Has Empty?"=w54:bool)
          n45 = Or(x=w55, y=w54) -> (x .or. y?=w53:bool)
          n46 = Not Or(1:w53, 2:w36) -> (0:w34:bool)
          n47 = case shown="True" w34 {
            tunnel: [T31."Settings" ("Tab Control") T28."Pressure/Temperature/Offsets" ("Tab Control")] -> w45
            frame False {
              # "Auto Switch to Settings Tab"
            }
            frame True {
              w61 = T29."Disabled and Grayed Out" ("Disabled")
              # "All Settings are valid!"
              n48 = property on="Input" class="Clust (strict)"("DisabledEnum"=w61) -> ()  [unwired: 2 in, 2 out]
              n49 = property on="Output" class="Clust (strict)"("DisabledEnum"=w61) -> ()  [unwired: 2 in, 2 out]
              n50 = property on="Safety" class="Clust (strict)"("DisabledEnum"=T29."Enabled" ("Disabled")) -> ()  [unwired: 2 in, 2 out]
            }
          }
          n51 = Not(x=w34) -> (.not. x?=w52:bool)
          n52 = Not(x=w34) -> (.not. x?=w35:bool)
          n53 = property on="System Running" class="Bool (strict)"("Value"=w34, "Blinking"=w35) -> ()  [unwired: 2 in, 2 out]
          n54 = call "Display Message to User5"("Enable"=w52, "Message"="Every line needs a Physical Channel!") -> ("OK"=w50:bool)  [unwired: 8 in, 1 out]
          n55 = Stop(stop? (T)=w50) -> ()
          n56 = control-ref of="Commit Settings"() -> (w44:refnum<vi>)
          n57 = property class="Bool (strict)"(reference=w44, "Value"=FALSE ("Commit Settings")) -> ()  [unwired: 1 in, 2 out]
          n58 = property on="Tab Control" class="TabCtl (strict)"("Value"=w45) -> ()  [unwired: 2 in, 2 out]
        }
        frame Disabled {
        }
      }
      n59 = disable-structure shown="Enabled" {
        frame Enabled {
          w22 = "msgQueue" ("name (unnamed)")
          # "Error/Warning Message Queue"
          n60 = Obtain Queue(name (unnamed)=w22, element data type=w22) -> ()  [unwired: 3 in, 3 out]
        }
        frame Disabled {
        }
      }
      n61 = disable-structure shown="Enabled" {
        frame Disabled {
        }
        frame Enabled {
          # "Queue for determining Psat Offsets"
          n62 = Initialize Array(0.0 ("element"), 8 ("dimension size")) -> (w33:dbl[])
          n63 = Obtain Queue(name (unnamed)="autoOffsetPsatQueue", element data type=w33) -> (queue out=→"autoOffsetPsatQueue":refnum<queue>)  [unwired: 3 in, 2 out]
          n64 = Obtain Queue(name (unnamed)="dataQueue", element data type=dbl[][] [] ("appended array")) -> (queue out=→"dataQueue":refnum<queue>)  [unwired: 3 in, 2 out]
          n65 = Obtain Notifier(name (unnamed)="diode_data_transfer_notifier", notification data type=T11 {"Liquid Diodes"={0.0, 0.0}, "Liquid Intensity Ratio"=0.0, "Vapor Diode"={0.0, 0.0}, "Vapor Intensity Ratio"=0.0, "TS Window 1 Temperatures"={"Average"=0.0, "T Sat [C]"=0.0}} ("Diode Charts")) -> (notifier out=→"notifier out":refnum<notifier>)  [unwired: 2 in, 2 out]
        }
      }
    }
    frame #2 {
      w116 = "WindowPowerBack" ("Channel Name")
      w117 = "WindowPowerFront" ("Channel Name")
      w138 = "Power" ("Channel Name")
      w155 = 10178 items=["Finite Samples"=10178, "Continuous Samples"=10123, "Hardware Timed Single Point"=12522] ("sample mode")
      w151 = 2 ("samples per channel")
      w160 = string[] ["MegaTankPressure", "MegaTankTemperature", "SeparatorPressure", "SeparatorTemperature", "LiquidInletPressure", "LiquidInletTemperature", "VaporInletPressure", "VaporInletTemperature", "VaporInletPressure", "VaporInletTemperature", "TSWindow1AbsolutePressure", "Toutlet", "UpperDevSectionPressure", "UpperDevSectionTemperature", "LowerDevSectionPressure", "PGinlet-MixingTeePressure", "VaporLinePitotdP", "AtmosphericPressure"] ("Array")
      w171 = 10123 items=["Finite Samples"=10178, "Continuous Samples"=10123, "Hardware Timed Single Point"=12522]  # sample mode
      w169 = 2000.0  # sampling rate
      w170 = 200  # number of samples
      # "Build labels for data logging"
      n66 = disable-structure shown="Enabled" {
        frame Enabled {
          n67 = global write "Stop_Global_Variable.vi" "Stop"("Stop") -> ()
        }
        frame Disabled {
        }
      }
      n68 = call "input_channel_task.vi"() -> ("error out"=w156:errorcluster, "Active Analog Channel-Data Packages"=w166:T38[], "task out"=w157:refnum<k21>)  [unwired: 9 in]
      n69 = call-poly <vilib>:"DAQmx Timing.vi"("task/channels in"=w157, "sample mode"=w155, "samples per channel"=w151, "rate"=1000.0, "error in"=w156) -> ("task out"=w153:refnum<k21>, "error out"=w152:errorcluster)  [unwired: 9 in]
      n70 = for {
        tunnel: w166 -> [w645] mode=indexing
        tunnel: [w644] -> w132 mode=indexing
        tunnel: [w642] -> w163 mode=indexing
        # "Compile list of channel data"
        n71 = Unbundle By Name(w645) -> ("Analog Data"=w644:T40, "Analog Data.Label"=w640:string, "Analog Data.Offset"=w643:dbl, "Analog Input Channel.Output Unit"=w641:T41)
        n72 = Bundle("Label"=w640, "Offset"=w643, "Output Unit"=w641) -> (w642:T42)  [unwired: 1 in]
      }
      n73 = call-poly <vilib>:"DAQmx Read.vi"("task/channels in"=w153, "number of samples per channel"=w151, "error in"=w152) -> ("task out"=w150:refnum<k21>, "data"=w133:waveform(dbl)[], "error out"=w149:errorcluster)  [unwired: 10 in]
      n74 = call <vilib>:"DAQmx Stop Task.vi"("task/channels in"=w150, "error in"=w149) -> ("task out"=w147:refnum<k21>, "error out"=w148:errorcluster)  [unwired: 12 in]
      n75 = property on="Offsets" class="Arr (strict)"("Val(Sgnl)"=w163) -> (error out=w135:errorcluster)  [unwired: 2 in, 1 out]
      n76 = Bundle By Name(cluster=T32 {"Channel Name"="", "Label"="", "Offset"=0.0, "Raw"=[], "Processed"=[], "Converted"=[], "Average"=0.0} ("Add-on Data"), "Channel Name"=w138, "Label"=w138) -> (w139:T32)
      n77 = Bundle By Name(cluster=T32 {"Channel Name"="", "Label"="", "Offset"=0.0, "Raw"=[], "Processed"=[], "Converted"=[], "Average"=0.0} ("Add-on Data"), "Channel Name"=w116, "Label"=w116) -> (w112:T32)
      n78 = Bundle By Name(cluster=T32 {"Channel Name"="", "Label"="", "Offset"=0.0, "Raw"=[], "Processed"=[], "Converted"=[], "Average"=0.0} ("Add-on Data"), "Channel Name"=w117, "Label"=w117) -> (w113:T32)
      n79 = call "data_processor.vi"("Active Analog Data Packages In"=w132, "data"=w133, "error in"=w135) -> ("Analog Data Array"=w137:T40[], "error out"=w136:errorcluster)  [unwired: 9 in, 2 out]
      n80 = call-poly <vilib>:"DAQmx Timing.vi"("task/channels in"=w147, "sample mode"=w171, "samples per channel"=w170, "rate"=w169, "error in"=w148) -> ("task out"=w97:refnum<k21>, "error out"=w94:errorcluster)  [unwired: 9 in]
      n81 = call "add_entry.vi"("Active Analog Data In"=w137, "Add-on Data"=w139, "error in"=w136) -> ("Active Analog Data Out"=w123:T40[], "error out"=w122:errorcluster)  [unwired: 11 in]
      n82 = property on="Sampling\nFrequency" class="DigNum (strict)"(error in=w94, "Value"=w169) -> (error out=w98:errorcluster)  [unwired: 1 in, 1 out]
      n83 = call "add_entry.vi"("Active Analog Data In"=w123, "Add-on Data"=w113, "error in"=w122) -> ("Active Analog Data Out"=w121:T40[], "error out"=w120:errorcluster)  [unwired: 11 in]
      n84 = property class="DAQmx Timing"(reference=w97, error in=w94) -> (reference out=w96:refnum<k21>, error out=w95:errorcluster, "SampClk.MaxRate"=w93:dbl)
      n85 = call "add_entry.vi"("Active Analog Data In"=w121, "Add-on Data"=w112, "error in"=w120) -> ("Active Analog Data Out"=w119:T40[], "error out"=w118:errorcluster)  [unwired: 11 in]
      n86 = property on="Offset Parameters" class="Clust (strict)"(error in=w95) -> (error out=w110:errorcluster, "Value"=w111:T4)  [unwired: 1 in, 1 out]
      n87 = call "find_label_indicies.vi"("error in"=w118, "Array"=T33[] [{"Label Array"=["VenturidP", "PGminiPressure", "PGminiTemperature"]}, {"Label Array"=["AtmosphericPressure"]}, {"Label Array"=["MegaTankPressure", "MegaTankTemperature", "SeparatorPressure", "SeparatorTemperature", "LiquidInletPressure", "LiquidInletTemperature", "VaporInletPressure", "VaporInletTemperature", "VaporInletPressure", "VaporInletTemperature", "TSWindow1AbsolutePressure", "Toutlet", "UpperDevSectionPressure", "UpperDevSectionTemperature", "LowerDevSectionPressure", "UpperDevSectionTemperature"]}, {"Label Array"=["VaporLineDensity", "LiquidLineDensity"]}, {"Label Array"=["VaporInletPressure", "LiquidMassFlow", "VaporMassFlow", "LiquidInletTemperature", "SeparatorTemperature"]}, {"Label Array"=["PGAbsolutePressure", "PGVaporTemperature", "PGLiquidTemperature", "PGSupplyTemperature", "Tinlet", "Tsectwo", "TSWindow1AbsolutePressure", "TSWindow7AbsolutePressure", "Window1to4dP", "Window1to7dP", "Window1to7FastdP", "VenturidP", "DwyerdP", "Tsecthree", "Toutlet", "TSExteriorTemperature"]}, {"Label Array"=["LiquidMainDiode", "LiquidControlDiode", "VaporMainDiode", "VaporControlDiode", "TSExteriorTemperature", "TSWindow1AbsolutePressure"]}, {"Label Array"=["VaporMassFlow", "VaporLineDensity", "LiquidMassFlow", "LiquidLineDensity", "CameraVoltage"]}], "haystack"=w119) -> ("error out"=w134:errorcluster, "Indicies"=w165:T43[])  [unwired: 6 in, 1 out]
      n88 = property on="Offset Parameters" class="Clust (strict)"(error in=w110, "Val(Sgnl)"=w111) -> (error out=w109:errorcluster)  [unwired: 1 in, 1 out]
      n89 = property on="Sampling\nFrequency" class="DigNum (strict)"(error in=w98) -> ("Value"=w168:dbl)  [unwired: 1 in, 2 out]
      n90 = property on="Pulse Generator Offsets" class="Clust (strict)"(error in=w109) -> (error out=w106:errorcluster, "Value"=w108:T8)  [unwired: 1 in, 1 out]
      n91 = disable-structure shown="Disabled" {
        frame Disabled {
          n92 = local read "notifier out"() -> (w646:refnum<notifier>)
          n93 = case shown="\"Network Steams\"" enum16{"Network Steams", "Datasocket", "Serial"}."Network Steams" {
            tunnel: w646 -> [_ _ w649]
            tunnel: [_ _ w648] -> _
            frame Default {
            }
            frame "Datasocket" {
            }
            frame "Network Steams" {
              w658 = T44 0 items=["allocate as needed", "pre-allocate"] ("element allocation mode")
              n94 = local read "Output"() -> (w662:T19)
              n95 = Unbundle By Name(w662) -> ("Diode Communication.URL"=w661:string)
              n96 = Create Network Stream Writer Endpoint(5:5000 ("timeout in ms (-1)"), 6:w658, 7:1 ("writer buffer size"), 9:T11 {"Liquid Diodes"={0.0, 0.0}, "Liquid Intensity Ratio"=0.0, "Vapor Diode"={0.0, 0.0}, "Vapor Intensity Ratio"=0.0, "TS Window 1 Temperatures"={"Average"=0.0, "T Sat [C]"=0.0}} ("Diode Charts"), 10:w661, 11:"mfval_control" ("writer name")) -> (0:w650:errorcluster, 3:w651:refnum<k21>)  [unwired: 1 in]
              n97 = while {
                tunnel: w649 -> [w670]
                tunnel: w651 -> [w673]
                tunnel: [w675] -> w653
                tunnel: w650 -> [w672]
                tunnel: [w674] -> w652
                stop <- w666 stop-if-true
                n98 = Wait on Notification(notifier=w670, ignore previous (F)=TRUE, error in (no error)=w672) -> (notification=w668:T11, timed out?=w667:bool, error out=w671:errorcluster)  [unwired: 1 in, 1 out]
                n99 = case shown="False" w667 {
                  tunnel: 80 ("timeout ms (-1)") -> [w683 _]
                  tunnel: [w682 w686] -> w675
                  tunnel: [w681 w685] -> w674
                  tunnel: w673 -> [w680 w686]
                  tunnel: [w679 FALSE] -> w665
                  tunnel: w671 -> [w678 w685]
                  tunnel: w668 -> [w677 _]
                  frame False {
                    n100 = shared-variable-write(w680, w678, w677, w683) -> (w682:refnum<k21>, w681:errorcluster, w679:bool)
                  }
                  frame True {
                  }
                }
                n101 = local read "Stop"() -> (w664:bool)
                n102 = Or(x=w665, y=w664) -> (x .or. y?=w666:bool)
              }
              n103 = Flush Stream(8:w652, 9:100 ("timeout in ms (-1)"), 11:w653) -> (0:w655:errorcluster, 3:w654:refnum<k21>)  [unwired: 1 in, 1 out]
              n104 = Destroy Stream Endpoint(8:w655, 11:w654) -> (0:w648:errorcluster)
            }
          }
        }
        frame Enabled {
        }
      }
      n105 = Get Date/Time In Seconds "Start Time\nIn Seconds"() -> (seconds since 1Jan1904=w172:timestamp)
      "start time" <- w172
      n106 = Tick Count (ms)() -> (millisecond timer value=w177:u32)
      n107 = property on="Pulse Generator Offsets" class="Clust (strict)"(error in=w106, "Val(Sgnl)"=w108) -> (error out=w107:errorcluster)  [unwired: 1 in, 1 out]
      n108 = call "build_labels.vi"("Analog Data Array In"=w119) -> ("Labels"=w142:string[][], "Label Indicies"=w141:i32[])  [unwired: 9 in]
      n109 = local read "start time"() -> (w167:timestamp)
      n110 = property on="Offsets" class="Arr (strict)"(error in=w134) -> ("Value"=w162:T27)  [unwired: 1 in, 2 out]
      n111 = property on="Data Labels" class="Arr (strict)"("Value"=w142) -> ()  [unwired: 2 in, 2 out]
      n112 = call <vilib>:"DAQmx Start Task.vi"("task/channels in"=w96, "error in"=w107) -> ("task out"=w158:refnum<k21>, "error out"=w91:errorcluster)  [unwired: 12 in]
      n113 = disable-structure shown="Enabled" {
        frame Disabled {
        }
        frame Enabled {
          # "Test Section Window Heater Safety Trigger"
          n114 = control-ref of="Tinlet"() -> (w775:refnum<vi>)
          n115 = control-ref of="Tsectwo"() -> (w774:refnum<vi>)
          n116 = control-ref of="Tsecthree"() -> (w772:refnum<vi>)
          n117 = control-ref of="Toutlet"() -> (w773:refnum<vi>)
          n118 = control-ref of="Vapor Flow rate [g/s]"() -> (w776:refnum<vi>)
          n119 = control-ref of="Liquid Flow rate [g/s]"() -> (w777:refnum<vi>)
          n120 = control-ref of="Stop"() -> (w771:refnum<vi>)
          n121 = control-ref of="Window Heater Switch"() -> (w779:refnum<vi>)
          n122 = control-ref of="Safety Trigger"() -> (w780:refnum<vi>)
          n123 = control-ref of="Maximum Test Section Temperature"() -> (w769:refnum<vi>)
          n124 = control-ref of="Minimum Test Section Mass Flow"() -> (w778:refnum<vi>)
          n125 = Build Array(w775, w774, w772, w773) -> (w770:refnum<vi>[])
          n126 = call "windows_heater_safety.vi"("Maximum Test Section Temperature"=w769, "Stop!"=w771, "Test Section Temperatures"=w770, "Minimum Flow Rate Refnum"=w778, "Liquid Flow Rate Refnum"=w777, "Vapor Flow Rate Refnum"=w776, "Safety Trigger Refnum"=w780, "Switch Refnum"=w779) -> ()  [unwired: 4 in]
        }
      }
      n127 = disable-structure shown="Enabled" {
        frame Disabled {
        }
        frame Enabled {
          # "Test Section Window Heater Switch"
          n128 = local read "Output"() -> (w768:T19)
          n129 = Unbundle By Name(w768) -> ("Window Heaters Physical Channels"=w765:T17)
          n130 = control-ref of="Reset PS Error"() -> (w761:refnum<vi>)
          n131 = property on="Front Readout" class="Clust (strict)"() -> ("Controls[]"=w764:refnum<vi>[])  [unwired: 2 in, 2 out]
          n132 = property on="Rear Readout" class="Clust (strict)"() -> ("Controls[]"=w763:refnum<vi>[])  [unwired: 2 in, 2 out]
          n133 = control-ref of="Window Heater Switch"() -> (w767:refnum<vi>)
          n134 = control-ref of="Stop"() -> (w766:refnum<vi>)
          n135 = Build Array(w764, w763) -> (w762:refnum<vi>[][])
          n136 = call "windows_heater.vi"("Power supply controls"=w762, "Window Heaters Physical Channels"=w765, "Switch Refnum"=w767, "Stop! Refnum"=w766, "Reset PS Error Refnum"=w761) -> ()  [unwired: 1 in]
        }
      }
      n137 = disable-structure shown="Enabled" {
        frame Enabled {
          # "Pulse Generator Safety Triggers"
          n138 = local read "Input"() -> (w817:T14)
          n139 = control-ref of="Float 1"() -> (w833:refnum<vi>)
          n140 = control-ref of="Float 2"() -> (w831:refnum<vi>)
          n141 = control-ref of="Float 3"() -> (w830:refnum<vi>)
          n142 = control-ref of="Float 4"() -> (w832:refnum<vi>)
          n143 = control-ref of="Float 5"() -> (w820:refnum<vi>)
          n144 = Unbundle By Name(w817) -> ("Float Switch Line Mode"=w816:bool)
          n145 = Unbundle By Name(w817) -> ("Float Switch Physical Channels"=w819:T13)
          n146 = Build Array(w833, w831, w830, w832, w820) -> (w829:refnum<vi>[])
          n147 = control-ref of="Heater ON?"() -> (w826:refnum<vi>)
          n148 = control-ref of="Stop"() -> (w827:refnum<vi>)
          n149 = control-ref of="Pulse Generator"() -> (w828:refnum<vi>)
          n150 = control-ref of="Absolute Pulse Generator Pressure Limit"() -> (w824:refnum<vi>)
          n151 = control-ref of="Absolute Pulse Generator Temperature Limit"() -> (w822:refnum<vi>)
          n152 = control-ref of="Seconds Allowed Pulse Generator Excess Pressure"() -> (w823:refnum<vi>)
          n153 = control-ref of="Liquid Temperature"() -> (w821:refnum<vi>)
          n154 = control-ref of="PG Abs Pressure"() -> (w825:refnum<vi>)
          n155 = Cluster To Array(cluster=w819) -> (array=w818:tag[])
          n156 = call "float_switch_check.vi"("Temperature Refnum"=w821, "Heater Refnum"=w826, "Abs Pressure Refnum"=w825, "InvertLines"=w816, "Abs Temperature Limit Refnum"=w822, "Timeout Refnum"=w823, "Abs Pressure Limit Refnum"=w824, "STOP! Refnum"=w827, "Pulse Generator Slide Refnum"=w828, "Float Indicator Refnum"=w829, "lines array"=w818) -> ()
        }
        frame Disabled {
        }
      }
      n157 = while {
        tunnel: w158 -> [w560]
        shift-right: [w553] -> _
        shift-left: w177 -> [w554]
        tunnel: w172 -> [w556]
        tunnel: [w464] -> w159
        shift-right: [w549] -> _
        shift-left: w168 -> [w550]
        shift-right: [w547] -> _
        shift-left: w170 -> [w548]
        tunnel: w167 -> [w546]
        shift-right: [w544] -> _
        shift-left: w119 -> [w508]
        tunnel: w165 -> [w531]
        shift-right: [w510] -> _
        shift-left: w162 -> [w545]
        tunnel: w141 -> [w516]
        tunnel: w93 -> [w472]
        shift-right: [w466] -> w92
        shift-left: w91 -> [w461]
        i -> [w558]
        stop <- w559 stop-if-true
        n158 = local read "Stop"() -> (w559:bool)
        n159 = Get Date/Time In Seconds "Iteration\nStart Time"() -> (seconds since 1Jan1904=w557:timestamp)
        "Time Stamp" <- w557
        n160 = call "loop_time.vi"("previous timer value"=w554) -> ("millisecond timer value"=w553:u32, "Loop Time [ms]"=→"Loop Time [ms]":u32)
        n161 = Subtract(x=w557, y=w556) -> (x-y=→"Seconds Since\nSession Start":dbl)
        n162 = call-poly <vilib>:"DAQmx Read.vi"("task/channels in"=w560, "number of samples per channel"=w548, "error in"=w461) -> ("task out"=w474:refnum<k21>, "data"=w507:waveform(dbl)[], "error out"=w481:errorcluster)  [unwired: 10 in]
        n163 = call "data_processor.vi"("Active Analog Data Packages In"=w508, "start time"=w546, "data"=w507, "error in"=w481) -> ("Analog Data Array"=w503:T40[], "timestamp"=w530:dbl[], "Number of Points"=w493:i32, "error out"=w529:errorcluster)  [unwired: 8 in]
        n164 = property on="Pressure/Temperature/Mixture Properties" class="Clust (strict)"(error in=w481) -> (error out=w469:errorcluster, "Value"=w532:T3)  [unwired: 1 in, 1 out]
        n165 = call "data_distributor_naive.vi"("Analog Data Array In"=w503, "Indicies"=w531, "error in"=w529) -> ("Pulse Generator Charts"=w528:T10, "Diode Charts"=w527:T11, "Measurements Data"=w514:T9, "Pressure/Temperature/Mixture Properties"=w515:T3, "Vapor Flow"=w492:cluster{"Average":dbl, "Average":dbl}, "Liquid Flow"=w491:cluster{"Average":dbl, "Average":dbl}, "CameraVoltage"=→"Camera Voltage":dbl[], "error out"=w526:errorcluster)  [unwired: 5 in]
        n166 = local read "autoOffsetPsatQueue"() -> (w536:refnum<queue>)
        n167 = local write "Pulse Generator Charts"(w528) -> ()
        n168 = local write "Diode Charts"(w527) -> ()
        n169 = property on="Flow" class="Clust (strict)"("Value"=w491) -> ()  [unwired: 2 in, 2 out]
        n170 = property on="Flow" class="Clust (strict)"("Value"=w492) -> ()  [unwired: 2 in, 2 out]
        n171 = control-ref of="Auto Offset"() -> (w535:refnum<vi>)
        n172 = property on="Sampling\nFrequency" class="DigNum (strict)"() -> ("Value"=w473:dbl)  [unwired: 2 in, 2 out]
        n173 = control-ref of="Auto Offset Progress"() -> (w533:refnum<vi>)
        n174 = property on="Vapor PID Control" class="Clust (strict)"(error in=w481) -> (error out=w479:errorcluster, "Value"=w482:T45)  [unwired: 1 in, 1 out]
        n175 = property on="Liquid PID Control" class="Clust (strict)"(error in=w481) -> (error out=w478:errorcluster, "Value"=w480:T45)  [unwired: 1 in, 1 out]
        n176 = call "brians_diode_screen.vi"("Diode Charts In"=w527) -> ()
        n177 = local write "Measurements Data"(w514) -> ()
        n178 = local write "Pressure/Temperature/Mixture Properties"(w515) -> ()
        n179 = property on="Power [W]" class="DigNum (strict)"(error in=w526) -> (error out=w505:errorcluster, "Value"=w512:dbl)  [unwired: 1 in, 1 out]
        n180 = call "enqueue_pressure_auto_offset.vi"("autoOffsetPsatQueue"=w536, "# to average"=30.0, "Auto Offset"=w535, "Pressure/Temperature/Mixture Properties"=w532, "Auto Offset ProgressBar"=w533) -> ()
        n181 = In Range and Coerce(upper limit=w472, x=w473, lower limit=1.0) -> (coerced(x)=w470:dbl)  [unwired: 1 out]
        n182 = property on="Sampling\nFrequency" class="DigNum (strict)"("Value"=w470) -> ()  [unwired: 2 in, 2 out]
        n183 = Merge Errors(w478, w479, w469) -> (w475:errorcluster)
        n184 = property on="Front Power" class="DigNum (strict)"(error in=w505) -> (error out=w504:errorcluster, "Value"=w495:dbl)  [unwired: 1 in, 1 out]
        n185 = property on="Rear Power" class="DigNum (strict)"(error in=w504) -> (error out=w498:errorcluster, "Value"=w494:dbl)  [unwired: 1 in, 1 out]
        n186 = local read "Data Saving Parameters"() -> (w522:T1)
        n187 = Unbundle By Name(w482) -> ("Valve Open Voltage [V]"=w489:dbl, "Valve On/Off"=w490:bool)
        n188 = Unbundle By Name(w480) -> ("Valve Open Voltage [V]"=w485:dbl, "Valve On/Off"=w486:bool)
        n189 = Unbundle By Name(w480) -> ("Flow Set Point [g/s]"=w542:dbl, "Flow.Flow rate [g/s]"=w541:dbl)
        n190 = Unbundle By Name(w482) -> ("Flow Set Point [g/s]"=w540:dbl, "Flow.Flow rate [g/s]"=w539:dbl)
        n191 = call "edit_entry.vi"("Average"=w495, "error in"=w498, "size(s)"=w493, "Label"="WindowPowerFront", "Active Analog Data In"=w503) -> ("error out"=w497:errorcluster, "Active Analog Data Out"=w502:T40[])  [unwired: 4 in, 1 out]
        n192 = call "edit_entry.vi"("Average"=w494, "error in"=w497, "size(s)"=w493, "Label"="WindowPowerBack", "Active Analog Data In"=w502) -> ("error out"=w496:errorcluster, "Active Analog Data Out"=w501:T40[])  [unwired: 4 in, 1 out]
        n193 = Unbundle By Name(w522) -> ("Sampling\nFrequency"=w524:dbl, "Recording Duration [s]"=w523:dbl)
        n194 = Bundle("Flow Set Point [g/s]"=w540, "Flow rate [g/s]"=w539) -> (→"Vapor Mass Flow Rate":T6)  [unwired: 1 in]
        n195 = Bundle("Flow Set Point [g/s]"=w542, "Flow rate [g/s]"=w541) -> (→"Liquid Mass Flow Rate":T6)  [unwired: 1 in]
        n196 = Select(t=w489, s=w490, f=0.0) -> (s? t:f=w484:dbl)
        n197 = Select(t=w485, s=w486, f=0.0) -> (s? t:f=w483:dbl)
        n198 = local read "dataQueue"() -> (w521:refnum<queue>)
        n199 = control-ref of="Record Data"() -> (w520:refnum<vi>)
        n200 = control-ref of="Data Recording Progress"() -> (w519:refnum<vi>)
        n201 = Build Array(w484, w483) -> (→"Valve Voltage Output":dbl[])
        n202 = call "edit_entry.vi"("Average"=w512, "error in"=w496, "size(s)"=w493, "Label"="Power", "Active Analog Data In"=w501) -> ("error out"=w525:errorcluster, "Active Analog Data Out"=w511:T40[])  [unwired: 4 in, 1 out]
        n203 = Multiply(x=w524, y=w523) -> (x*y=w518:dbl)
        n204 = call "enqueue_data.vi"("Active Analog Data In"=w511, "Label indicies In"=w516, "timestamp"=w530, "# of Samples"=w518, "error in"=w525, "data Queue"=w521, "Record dP Data"=w520, "dP Recording Progress"=w519) -> ("error out"=w509:errorcluster)  [unwired: 7 in]
        n205 = property on="Offsets" class="Arr (strict)"(error in=w509) -> (error out=w476:errorcluster, "Value"=w510:T27)  [unwired: 1 in, 1 out]
        n206 = Equal?(x=w550, y=w470) -> (x = y?=w551:bool)
        n207 = Merge Errors(w475, w476) -> (w477:errorcluster)
        n208 = case shown="False" w551 {
          tunnel: w550 -> [_ w599]
          tunnel: [w591 w599] -> w549
          tunnel: w470 -> [w591 _]
          tunnel: w474 -> [w595 w598]
          tunnel: w477 -> [w594 w596]
          tunnel: [w586 w598] -> w462
          tunnel: w548 -> [_ w597]
          tunnel: [w587 w597] -> w547
          tunnel: [w585 w596] -> w463
          frame False {
            n209 = call <vilib>:"DAQmx Stop Task.vi"("task/channels in"=w595, "error in"=w594) -> ("task out"=w593:refnum<k21>, "error out"=w592:errorcluster)  [unwired: 12 in]
            n210 = Divide(x=w591, y=10.0) -> (x/y=w587:dbl)
            n211 = property class="DAQmx Timing"(reference=w593, error in=w592, "SampClk.Rate"=w591, "SampQuant.SampPerChan"=w587) -> (reference out=w589:refnum<k21>, error out=w588:errorcluster)
            n212 = call <vilib>:"DAQmx Start Task.vi"("task/channels in"=w589, "error in"=w588) -> ("task out"=w586:refnum<k21>, "error out"=w585:errorcluster)  [unwired: 12 in]
          }
          frame True {
          }
        }
        n213 = Not Equal?(x=w510, y=w545) -> (x != y?=w517:bool)
        n214 = case shown="True" w517 {
          tunnel: w511 -> [w569 w570]
          tunnel: [w569 w571] -> w544
          frame False {
          }
          frame True {
            n215 = for {
              tunnel: "Offsets" -> [w574]
              tunnel: [w579] -> w571 mode=indexing
              tunnel: w570 -> [w578] mode=indexing
              i -> [w575]
              n216 = Array Size(array=w574) -> (size(s)=w577:i32)
              n217 = Index Array(array=w574, index=w575) -> (element=w573:T46)
              n218 = Less?(x=w575, y=w577) -> (x < y?=w576:bool)
              n219 = case shown="True" w576 {
                tunnel: [w580 w584] -> w579
                tunnel: w578 -> [w580 w582]
                tunnel: w573 -> [_ w581]
                frame False {
                }
                frame True {
                  n220 = Unbundle By Name(w581) -> ("Offset"=w583:dbl)
                  n221 = Bundle By Name(cluster=w582, "Offset"=w583) -> (w584:T40)
                }
              }
            }
          }
        }
        n222 = call <vilib>:"Clear Errors.vi"("error in (no error)"=w463, "specific error code to clear (0: all)"=-200279 ("error codes")) -> ("error out"=w467:errorcluster, "specific error cleared?"=w468:bool)  [unwired: 4 in]
        n223 = property on="Buffer Overflow" class="Bool (strict)"("Val(Sgnl)"=w468) -> ()  [unwired: 2 in, 2 out]
        n224 = case shown="True" w468 {
          tunnel: w467 -> [w562 w568]
          tunnel: [w562 w566] -> w466
          tunnel: [w561 w564] -> w464
          tunnel: w462 -> [w561 w563]
          frame False {
          }
          frame True {
            n225 = call <vilib>:"DAQmx Stop Task.vi"("task/channels in"=w563, "error in"=w568) -> ("task out"=w565:refnum<k21>, "error out"=w567:errorcluster)  [unwired: 12 in]
            n226 = call <vilib>:"DAQmx Start Task.vi"("task/channels in"=w565, "error in"=w567) -> ("task out"=w564:refnum<k21>, "error out"=w566:errorcluster)  [unwired: 12 in]
          }
        }
        "# of Datasets Processed" <- w558
      }
      n227 = while {
        tunnel: w119 -> [w410]
        stop <- w411 stop-if-true
        n228 = event shown="[1] \"Generate MATLAB Parsing Script\": Value Change" {
          selector: _ -> [_ _]
          dyn-events: _ -> [_ _]
          timeout: _ -> [_ _]
          tunnel: [TRUE _] -> w411
          tunnel: w410 -> [_ w413]
          event Timeout; "Stop": Value Change {
            n229 = event-data() -> ()  [unwired: 1 in, 3 out]
          }
          event "Generate MATLAB Parsing Script": Value Change {
            n230 = event-data() -> ("NewVal"=w414:bool)  [unwired: 1 in]
            n231 = case shown="True" w414 {
              tunnel: w413 -> [_ w417]
              frame False {
              }
              frame True {
                n232 = property on="Data Folder" class="Path"() -> ("Value"=w416:path)  [unwired: 2 in, 2 out]
                n233 = call "File Dialog"("start path"=w416) -> ("selected path"=w415:path)  [unwired: 11 in, 3 out]
                n234 = call "build_labels.vi"("MATLAB File Directory"=w415, "Save MATLAB Parser?"=TRUE, "Analog Data Array In"=w417) -> ()  [unwired: 7 in, 2 out]
              }
            }
          }
        }
      }
      n235 = disable-structure shown="Enabled" {
        frame Disabled {
        }
        frame Enabled {
          w799 = T47 {"Start Pulse"=refnum, "Stop Pulse"=refnum, "Heaters"=refnum, "Counter"=refnum, "Start Frequency (Hz)"=refnum, "Pulse Generator Active"=refnum, "Stepper Motor Direction"=refnum, "Ramp Duration"=refnum, "Direction Line"=refnum, "1000-1 Line"=refnum, "1000-2 Line"=refnum, "1000-3 Line"=refnum, "500-1 Line"=refnum, "250-1 Line"=refnum, "1000-1"=refnum, "1000-2"=refnum, "1000-3"=refnum, "500-1"=refnum, "250-1"=refnum, "150-1"=refnum, "Heater ON?"=refnum, "150-1 Line"=refnum, "Power"=refnum, "Steady Frequency (Hz)"=refnum, "Steady Duration "=refnum, "Pulse Mode"=refnum, "Frequency [Hz]"=refnum, "Avg % Open"=refnum, "Repetitions"=refnum, "+/- % Open"=refnum, "USB Controller"=refnum}  # Pulse Generator Control Refnums
          # "Controls Heaters and Stepper Motor, listens to stopping signals."
          n236 = control-ref of="USB controller"() -> (w782:refnum<vi>)
          n237 = control-ref of="Counter Line"() -> (w794:refnum<vi>)
          n238 = control-ref of="Direction Line"() -> (w792:refnum<vi>)
          n239 = control-ref of="1000W 1"() -> (w808:refnum<vi>)
          n240 = control-ref of="1000W 2"() -> (w814:refnum<vi>)
          n241 = control-ref of="1000W 3"() -> (w809:refnum<vi>)
          n242 = control-ref of="500W 1"() -> (w810:refnum<vi>)
          n243 = control-ref of="250W 1"() -> (w811:refnum<vi>)
          n244 = control-ref of="150W 1"() -> (w798:refnum<vi>)
          n245 = control-ref of="Start Pulse"() -> (w804:refnum<vi>)
          n246 = control-ref of="Stop Pulse"() -> (w803:refnum<vi>)
          n247 = control-ref of="Heaters"() -> (w800:refnum<vi>)
          n248 = control-ref of="Pulse Gen\nActive?"() -> (w791:refnum<vi>)
          n249 = control-ref of="Motor Dir"() -> (w801:refnum<vi>)
          n250 = control-ref of="Heater ON?"() -> (w807:refnum<vi>)
          n251 = control-ref of="1000-1"() -> (w813:refnum<vi>)
          n252 = control-ref of="1000-2"() -> (w812:refnum<vi>)
          n253 = control-ref of="1000-3"() -> (w815:refnum<vi>)
          n254 = control-ref of="500-1"() -> (w797:refnum<vi>)
          n255 = control-ref of="250-1"() -> (w796:refnum<vi>)
          n256 = control-ref of="150-1"() -> (w795:refnum<vi>)
          n257 = control-ref of="Frequency [Hz]"() -> (w786:refnum<vi>)
          n258 = control-ref of="Repetitions"() -> (w785:refnum<vi>)
          n259 = control-ref of="Pulse Mode"() -> (w784:refnum<vi>)
          n260 = control-ref of="+/- % Movement"() -> (w787:refnum<vi>)
          n261 = control-ref of="Average % Open"() -> (w783:refnum<vi>)
          n262 = control-ref of="Power [W]"() -> (w793:refnum<vi>)
          n263 = control-ref of="Steady Duration[s]"() -> (w788:refnum<vi>)
          n264 = control-ref of="Start Frequency [Hz]"() -> (w802:refnum<vi>)
          n265 = control-ref of="Ramp Duration [s]"() -> (w789:refnum<vi>)
          n266 = control-ref of="Steady Frequency [Hz]"() -> (w790:refnum<vi>)
          n267 = Bundle By Name(cluster=w799, "Start Pulse"=w804, "Stop Pulse"=w803, "Heaters"=w800, "Counter"=w794, "Start Frequency (Hz)"=w802, "Ramp Duration"=w789, "Steady Frequency (Hz)"=w790, "Steady Duration"=w788, "Pulse Generator Active"=w791, "Stepper Motor Direction"=w801, "Direction Line"=w792, "Heater ON?"=w807, "1000-1 Line"=w808, "1000-2 Line"=w814, "1000-3 Line"=w809, "500-1 Line"=w810, "250-1 Line"=w811, "150-1 Line"=w798, "1000-1"=w813, "1000-2"=w812, "1000-3"=w815, "500-1"=w797, "250-1"=w796, "150-1"=w795, "Power"=w793, "+/- % Open"=w787, "Frequency [Hz]"=w786, "Repetitions"=w785, "Pulse Mode"=w784, "Avg % Open"=w783, "USB Controller"=w782) -> (w805:T47)
          n268 = control-ref of="Stop"() -> (w806:refnum<vi>)
          n269 = call "pulse_generator_multiheater_continuous_driver_refnum.vi"("Stop! Refnum"=w806, "Pulse Generator Control Multiheater Refnums"=w805) -> ()  [unwired: 2 in]
        }
      }
      n270 = while {
        stop <- w834 stop-if-true
        # "Dequeue loop for auto offset function"
        n271 = event shown="[1] \"Auto Offset\": Value Change" {
          selector: _ -> [_ _]
          dyn-events: _ -> [_ _]
          timeout: _ -> [_ _]
          tunnel: [TRUE _] -> w834
          event Timeout; "Stop": Value Change {
            n272 = event-data() -> ()  [unwired: 1 in, 3 out]
          }
          event "Auto Offset": Value Change {
            n273 = event-data() -> ("NewVal"=w837:bool)  [unwired: 1 in]
            n274 = case shown="False" w837 {
              frame False {
                n275 = local read "autoOffsetPsatQueue"() -> (w865:refnum<queue>)
                n276 = Initialize Array(0.0 ("element"), 8 ("dimension size")) -> (w847:dbl[])
                n277 = while {
                  tunnel: w865 -> [w874]
                  shift-right: [w869] -> w864
                  shift-left: w847 -> [w870]
                  shift-right: [w866] -> w838
                  shift-left: 0 -> [w867]
                  stop <- w872 stop-if-true
                  n278 = Dequeue Element(queue=w874, timeout in ms (-1)=500) -> (element=w871:dbl[], timed out?=w873:bool)  [unwired: 1 in, 2 out]
                  n279 = case shown="False" w873 {
                    selector: w873 -> [_ w885]
                    tunnel: [w877 w885] -> w872
                    tunnel: w871 -> [w881 _]
                    tunnel: [w880 w884] -> w869
                    tunnel: w870 -> [w882 w884]
                    tunnel: w867 -> [w876 w883]
                    tunnel: [w875 w883] -> w866
                    frame False {
                      n280 = local read "Stop"() -> (w878:bool)
                      n281 = Add(x=w882, y=w881) -> (x+y=w880:dbl[])
                      n282 = Increment(x=w876) -> (x+1=w875:i32)
                      n283 = Or(x=w878, y=FALSE) -> (x .or. y?=w877:bool)
                    }
                    frame True {
                    }
                  }
                }
                n284 = property on="Offset Parameters" class="Clust (strict)"() -> ("Value"=w841:T4)  [unwired: 2 in, 2 out]
                n285 = Divide(x=w864, y=w838) -> (x/y=w863:dbl[])
                n286 = Unbundle By Name(w841) -> ("Mega Tank\nPressure"=w861:dbl, "Separator Pressure"=w860:dbl, "Liquid Inlet\nPressure"=w854:dbl, "Vapor Inlet\nPressure"=w859:dbl, "Vapor Inlet\nPressure"=w855:dbl, "Test Section\nPressure"=w858:dbl, "Upper Dev Section\nPressure"=w857:dbl, "Lower Dev Section\nPressure"=w842:dbl)
                n287 = Build Array(w861, w860, w854, w859, w855, w858, w857, w842) -> (w856:dbl[])
                n288 = Add(x=w863, y=w856) -> (x+y=w862:dbl[])
                n289 = Index Array(array=w862) -> (element #1=w853:dbl, element #2=w852:dbl, element #3=w851:dbl, element #4=w850:dbl, element #5=w846:dbl, element #6=w845:dbl, element #7=w844:dbl, element #8=w843:dbl)  [unwired: 8 in]
                n290 = Bundle By Name(cluster=w841, "Mega Tank\nPressure"=w853, "Separator Pressure"=w852, "Liquid Inlet\nPressure"=w851, "Vapor Inlet\nPressure"=w850, "Vapor Inlet\nPressure"=w846, "Test Section\nPressure"=w845, "Upper Dev Section\nPressure"=w844, "Lower Dev Section\nPressure"=w843) -> (w840:T4)
                n291 = property on="Offset Parameters" class="Clust (strict)"("Val(Sgnl)"=w840) -> ()  [unwired: 2 in, 2 out]
              }
              frame True {
                n292 = property on="Offset Parameters" class="Clust (strict)"("DisabledEnum"=T29."Disabled and Grayed Out" ("Disabled")) -> ()  [unwired: 2 in, 2 out]
              }
            }
            n293 = property on="Offset Parameters" class="Clust (strict)"("DisabledEnum"=T29."Enabled" ("Disabled")) -> ()  [unwired: 2 in, 2 out]
          }
        }
      }
      n294 = while {
        tunnel: [w612] -> w127
        tunnel: [w611] -> w126
        stop <- w613 continue-if-true
        n295 = property on="# of Datasets Processed" class="DigNum (strict)"() -> (error out=w612:errorcluster, "Value"=w615:i32)  [unwired: 2 in, 1 out]
        n296 = Less?(x=w615, y=1) -> (x < y?=w613:bool)
        n297 = local read "Offsets"() -> (w611:T27)
      }
      n298 = control-ref of="1000W 1 PID"() -> (w90:refnum<vi>)
      n299 = control-ref of="1000W 2 PID"() -> (w89:refnum<vi>)
      n300 = control-ref of="1000W 3 PID"() -> (w88:refnum<vi>)
      n301 = control-ref of="500W 1 PID"() -> (w87:refnum<vi>)
      n302 = control-ref of="250W 1 PID"() -> (w86:refnum<vi>)
      n303 = control-ref of="150W 1 PID"() -> (w85:refnum<vi>)
      n304 = control-ref of="1000-1"() -> (w84:refnum<vi>)
      n305 = control-ref of="1000-2"() -> (w83:refnum<vi>)
      n306 = control-ref of="1000-3"() -> (w82:refnum<vi>)
      n307 = control-ref of="500-1"() -> (w81:refnum<vi>)
      n308 = control-ref of="250-1"() -> (w80:refnum<vi>)
      n309 = control-ref of="150-1"() -> (w79:refnum<vi>)
      n310 = Array Size(array=w160) -> (size(s)=w161:i32)
      n311 = for {
        N: w161 -> [_]
        tunnel: w160 -> [w604] mode=indexing
        tunnel: w127 -> [_]
        tunnel: w126 -> [w605]
        tunnel: [w600] -> w128 mode=indexing
        n312 = for {
          tunnel: w605 -> [w610] mode=indexing
          tunnel: w604 -> [w608]
          tunnel: [w607] -> w602
          tunnel: [w606] -> w603
          i -> [w607]
          stop <- w606 stop-if-true
          n313 = Unbundle(w610) -> ("Channel"=w609:string)  [unwired: 2 out]
          n314 = Equal?(x=w609, y=w608) -> (x = y?=w606:bool)
        }
        n315 = Select(t=w602, s=w603, f=-1) -> (s? t:f=w600:i32)
      }
      n316 = for {
        tunnel: string[] ["PGAbsolutePressure", "VenturidP", "Window1to4dP", "Window1to7dP", "Window1to7FastdP", "TSWindow1AbsolutePressure", "TSWindow7AbsolutePressure", "DwyerdP"] ("Array") -> [w403] mode=indexing
        tunnel: w126 -> [w404]
        tunnel: [w399] -> w124 mode=indexing
        tunnel: w127 -> [_]
        n317 = for {
          tunnel: w404 -> [w409] mode=indexing
          tunnel: w403 -> [w407]
          tunnel: [w406] -> w401
          tunnel: [w405] -> w402
          i -> [w406]
          stop <- w405 stop-if-true
          n318 = Unbundle(w409) -> ("Channel"=w408:string)  [unwired: 2 out]
          n319 = Equal?(x=w408, y=w407) -> (x = y?=w405:bool)
        }
        n320 = Select(t=w401, s=w402, f=-1) -> (s? t:f=w399:i32)
      }
      n321 = Build Array(w84, w83, w82, w81, w80, w79) -> (w77:refnum<vi>[])
      n322 = Build Array(w90, w89, w88, w87, w86, w85) -> (w78:refnum<vi>[])
      n323 = while {
        tunnel: w78 -> [w214]
        tunnel: w77 -> [w213]
        stop <- w215 stop-if-true
        # "PG Pressure Controller"
        n324 = property on="PG Controller Switch" class="Bool (strict)"() -> ("Value"=w212:bool)  [unwired: 2 in, 2 out]
        n325 = local read "Stop"() -> (w215:bool)
        n326 = Wait (ms)(milliseconds to wait=u32 100) -> ()  [unwired: 1 out]
        n327 = case shown="True" w212 {
          tunnel: w214 -> [_ w218]
          tunnel: w213 -> [_ w217]
          frame False {
          }
          frame True {
            n328 = property on="PG Abs Pressure" class="DigNum (strict)"() -> ("Value"=w221:dbl)  [unwired: 2 in, 2 out]
            n329 = property on="Hysteresis" class="DigNum (strict)"() -> ("Value"=w219:dbl)  [unwired: 2 in, 2 out]
            n330 = property on="Setpoint [Pa]" class="DigNum (strict)"() -> ("Value"=w222:dbl)  [unwired: 2 in, 2 out]
            n331 = Subtract(x=w222, y=w221) -> (x-y=w220:dbl)
            n332 = Greater?(x=w220, y=w219) -> (0:w216:bool)
            n333 = case shown="False" w216 {
              tunnel: w218 -> [w223 w232]
              tunnel: w217 -> [w224 w231]
              frame False {
                # "Turn off selected heaters if false"
                n334 = for {
                  tunnel: w223 -> [w227] mode=indexing
                  tunnel: w224 -> [w226] mode=indexing
                  n335 = property class="Bool (strict)"(reference=w227) -> ("Value"=w225:bool)  [unwired: 1 in, 2 out]
                  n336 = case shown="True" w225 {
                    selector: w225 -> [_ w229]
                    tunnel: w226 -> [_ w230]
                    frame False {
                    }
                    frame True {
                      n337 = Not(x=w229) -> (.not. x?=w228:bool)
                      n338 = property class="Bool (strict)"(reference=w230, "Value"=w228) -> ()  [unwired: 1 in, 2 out]
                    }
                  }
                }
              }
              frame True {
                # "Turn on selected heaters if True."
                n339 = for {
                  tunnel: w232 -> [w235] mode=indexing
                  tunnel: w231 -> [w234] mode=indexing
                  n340 = property class="Bool (strict)"(reference=w235) -> ("Value"=w233:bool)  [unwired: 1 in, 2 out]
                  n341 = case shown="True" w233 {
                    selector: w233 -> [_ w236]
                    tunnel: w234 -> [_ w237]
                    frame False {
                    }
                    frame True {
                      n342 = property class="Bool (strict)"(reference=w237, "Value"=w236) -> ()  [unwired: 1 in, 2 out]
                    }
                  }
                }
              }
            }
          }
        }
      }
      n343 = while {
        tunnel: w128 -> [w617]
        tunnel: w124 -> [w616]
        stop <- w620 stop-if-true
        n344 = event shown="[2] \"Pulse Generator Offsets\": Value Change" {
          selector: _ -> [_ _ _]
          dyn-events: _ -> [_ _ _]
          timeout: _ -> [_ _ _]
          tunnel: [TRUE _ _] -> w618
          tunnel: w617 -> [_ w622 _]
          tunnel: w616 -> [_ _ w631]
          event Timeout; "Stop": Value Change {
            n345 = event-data() -> ()  [unwired: 1 in, 3 out]
          }
          event Value Change {
            n346 = event-data() -> ("NewVal"=w624:T4)  [unwired: 1 in]
            n347 = Cluster To Array(cluster=w624) -> (array=w623:dbl[])
            n348 = for {
              tunnel: w623 -> [w627] mode=indexing
              tunnel: w622 -> [w630] mode=indexing
              n349 = local read "Offsets"() -> (w628:T27)
              n350 = Index Array(array=w628, index=w630) -> (element=w629:T46)
              n351 = Bundle By Name(cluster=w629, "Offset"=w627) -> (w626:T46)
              n352 = Replace Array Subset(array=w628, new element=w626, index=w630) -> (w625:T27)
              n353 = local write "Offsets"(w625) -> ()
            }
          }
          event Value Change {
            n354 = event-data() -> ("NewVal"=w632:T8)  [unwired: 1 in]
            n355 = Cluster To Array(cluster=w632) -> (array=w633:dbl[])
            n356 = for {
              tunnel: w633 -> [w636] mode=indexing
              tunnel: w631 -> [w639] mode=indexing
              n357 = local read "Offsets"() -> (w637:T27)
              n358 = Index Array(array=w637, index=w639) -> (element=w638:T46)
              n359 = Bundle By Name(cluster=w638, "Offset"=w636) -> (w635:T46)
              n360 = Replace Array Subset(array=w637, new element=w635, index=w639) -> (w634:T27)
              n361 = local write "Offsets"(w634) -> ()
            }
          }
        }
        n362 = local read "Stop"() -> (w619:bool)
        n363 = Or(x=w618, y=w619) -> (x .or. y?=w620:bool)
      }
      n364 = while {
        stop <- w736 stop-if-true
        # "Updates Visual Loop Data Display (low priority)"
        n365 = local read "Measurements Data"() -> (w744:T9)
        n366 = local read "Pressure/Temperature/Mixture Properties"() -> (w760:T3)
        n367 = Unbundle By Name(w760) -> ("Component PTs"=w759:T48, "Ambient Pressure [Pa]"=w745:dbl)
        n368 = local read "Liquid PID Control"() -> (w732:T7)
        n369 = local read "Vapor PID Control"() -> (w731:T7)
        n370 = Wait (ms)(milliseconds to wait=u32 500) -> ()  [unwired: 1 out]
        n371 = Unbundle By Name(w744) -> ("PG Abs Pressure"=w743:dbl, "PG Mass Flow Rate"=w742:dbl, "Vapor Temperature"=w741:dbl, "Liquid Temperature"=w740:dbl, "W1-4 dP[Pa]"=w739:dbl, "W1-7 dP[Pa]"=w738:dbl)
        n372 = Unbundle By Name(w759) -> ("Liquid Tank P"=w757:dbl, "Liquid Tank T"=w756:dbl, "Separator P"=w755:dbl, "Separator T"=w754:dbl, "Liquid Inlet P"=w753:dbl, "Liquid Inlet T"=w752:dbl, "Vapor Tank P"=w751:dbl, "Vapor Tank T"=w750:dbl, "Vapor Inlet P"=w749:dbl, "Vapor Inlet T"=w748:dbl, "Upper Dev Section P"=w747:dbl, "Lower Dev Section P"=w746:dbl)
        n373 = Unbundle By Name(w731) -> ("Flow.Flow rate [g/s]"=w735:dbl)
        n374 = Unbundle By Name(w732) -> ("Flow.Flow rate [g/s]"=w734:dbl)
        n375 = local read "Visual Loop Display"() -> (w758:T5)
        n376 = Bundle By Name(cluster=w758, "LiqTkPres"=w757, "LiqTkTemp"=w756, "SepPres"=w755, "SepTemp"=w754, "LiqInPres"=w753, "LiqInTemp"=w752, "VpTkPres"=w751, "VpTkTemp"=w750, "VapInPres"=w749, "VapInTemp"=w748, "TSInPres"=w747, "TSInTemp"=w746, "TSPres"=w745, "PgPres"=w743, "PGMass"=w742, "PGVapTemp"=w741, "PGLiqTemp"=w740, "Win1-4dP"=w739, "Win1-7dP"=w738, "VpMass"=w735, "LiqMass"=w734) -> (→"Visual Loop Display":T5)
        n377 = local read "Stop"() -> (w736:bool)
      }
      n378 = local read "Output"() -> (w105:T19)
      n379 = local read "dataQueue"() -> (w173:refnum<queue>)
      n380 = Unbundle By Name(w105) -> ("PLC Communication.Remote IP"=w103:string, "PLC Communication.Remote Port"=w104:u16)
      n381 = while {
        tunnel: w173 -> [w956]
        tunnel: [w952] -> _
        stop <- w953 stop-if-true
        # "Dequeue loop of data logging"
        n382 = local read "Stop"() -> (w953:bool)
        n383 = Dequeue Element(queue=w956, timeout in ms (-1)=50) -> (queue out=w952:refnum<queue>, element=w954:dbl[][], timed out?=w951:bool)  [unwired: 1 in, 1 out]
        n384 = case shown="False" w951 {
          tunnel: w954 -> [w961 _]
          frame False {
            n385 = property on="Data Prefix" class="Str"() -> ("Value"=w959:string)  [unwired: 2 in, 2 out]
            n386 = property on="Data Index" class="DigNum (strict)"() -> ("Value"=w958:i32)  [unwired: 2 in, 2 out]
            n387 = property on="Data Folder" class="Path"() -> ("Value"=w960:path)  [unwired: 2 in, 2 out]
            n388 = local read "Data Labels"() -> (w957:string[][])
            n389 = call "write_data.vi"("Data Folder"=w960, "dP Data Prefix"=w959, "dP Data Index"=w958, "Data Labels"=w957, "dequeued data"=w961) -> ()  [unwired: 1 in]
          }
          frame True {
          }
        }
      }
      n390 = while {
        tunnel: w173 -> [w888]
        stop <- w887 stop-if-true
        # "Makes sure the path and daq settings cannot be changed while data is being recorded."
        n391 = event shown="[1] \"Data Saving Parameters.Record Data\": Value Change" {
          selector: _ -> [_ _]
          dyn-events: _ -> [_ _]
          timeout: _ -> [_ _]
          tunnel: w888 -> [_ w891]
          tunnel: [TRUE _] -> w887
          event Timeout; "Stop": Value Change {
            n392 = event-data() -> ()  [unwired: 1 in, 3 out]
          }
          event "Data Saving Parameters.Record Data": Value Change {
            n393 = event-data() -> ("NewVal"=w890:bool)  [unwired: 1 in]
            n394 = case shown="False" w890 {
              tunnel: w891 -> [w893 _]
              frame False {
                n395 = flat-sequence {
                  tunnel: w893 -> [w895]
                  tunnel: [w904] -> w892
                  tunnel: w892 -> [w928]
                  frame #0 {
                    n396 = while {
                      tunnel: w895 -> [w896]
                      stop <- w897 stop-if-true
                      n397 = Get Queue Status(queue=w896) -> (# elements in queue=w901:i32)  [unwired: 2 in, 7 out]
                      n398 = local read "Stop"() -> (w898:bool)
                      n399 = Equal?(x=0, y=w901) -> (x = y?=w899:bool)
                      n400 = Or(x=w899, y=w898) -> (x .or. y?=w897:bool)
                    }
                    n401 = property on="Record Data" class="Bool (strict)"("DisabledEnum"=T29."Disabled and Grayed Out" ("Disabled")) -> ()  [unwired: 2 in, 2 out]
                  }
                  frame #1 {
                    n402 = Wait (ms)(milliseconds to wait=u32 500) -> ()  [unwired: 1 out]
                  }
                  frame #2 {
                    w915 = T49 5 items=["User Home"=0, "User Desktop"=1, "User Documents"=2, "User Application Data"=3, "User Preferences"=4, "User Temporary"=5, "Public Documents"=6, "Public Application Data"=7, "Public Preferences"=8, "Public Cache"=13, "System Core Libraries"=9, "System Installed Libraries"=10, "Application Files"=11, "Boot Volume Root"=12] ("system directory type")
                    n403 = property on="Notes:" class="Str"() -> ("Value"=w905:string)  [unwired: 2 in, 2 out]
                    n404 = property on="Data Index" class="DigNum (strict)"() -> ("Value"=w923:i32)  [unwired: 2 in, 2 out]
                    n405 = property on="Data Prefix" class="Str"() -> ("Value"=w921:string)  [unwired: 2 in, 2 out]
                    n406 = property on="Data Index" class="DigNum (strict)"() -> ("Value"=w906:i32)  [unwired: 2 in, 2 out]
                    n407 = Format Into String(format string="%04d", w906) -> (resulting string=w908:string)  [unwired: 2 in, 1 out]
                    n408 = call <vilib>:"Get System Directory.vi"("system directory type"=w915) -> ("system directory"=w924:path)  [unwired: 10 in]
                    n409 = Format Into String(format string="%04d%s", initial string="mfval_temp_", w923, ".csv") -> (resulting string=w925:string)  [unwired: 1 in, 1 out]
                    n410 = Format Into String(format string="-%04d%s", initial string=w921, w906, ".csv") -> (resulting string=w920:string)  [unwired: 1 in, 1 out]
                    n411 = Bundle(cluster=T35 {"Entry Content"="", "File Number"=""} ("new element/subarray"), "Entry Content"=w908, "File Number"=w905) -> (w909:T35)
                    n412 = property on="Data Folder" class="Path"() -> ("Value"=w919:path)  [unwired: 2 in, 2 out]
                    n413 = Insert Into Array(array="Run Log", new element=w909) -> (w904:T22)  [unwired: 1 in]
                    n414 = Build Path(base path=w924, name or relative path=w925) -> (appended path=w922:path)
                    n415 = Build Path(base path=w919, name or relative path=w920) -> (appended path=w918:path)
                    n416 = Move(source path=w922, 9:TRUE ("overwrite (F)"), 10:w918) -> ()  [unwired: 2 in, 3 out]
                  }
                  frame #3 {
                    w933 = T29."Enabled" ("Disabled")
                    w934 = T29."Enabled" ("Disabled")
                    n417 = local write "Run Log"(w928) -> ()
                    n418 = property on="Data Index" class="DigNum (strict)"() -> (error out=w935:errorcluster, "Value"=w937:i32)  [unwired: 2 in, 1 out]
                    n419 = for {
                      tunnel: w928 -> [w939] mode=indexing
                      tunnel: [w938] -> w927 mode=indexing
                      n420 = Cluster To Array(cluster=w939) -> (array=w938:string[])
                    }
                    n421 = Increment(x=w937) -> (x+1=w936:i32)
                    n422 = property on="Data Index" class="DigNum (strict)"(error in=w935, "Value"=w936) -> ()  [unwired: 1 in, 2 out]
                    n423 = property on="Data Folder" class="Path"("DisabledEnum"=w934) -> ()  [unwired: 2 in, 2 out]
                    n424 = property on="Data Prefix" class="Str"("DisabledEnum"=w934) -> ()  [unwired: 2 in, 2 out]
                    n425 = property on="Data Folder" class="Path"() -> ("Value"=w931:path)  [unwired: 2 in, 2 out]
                    n426 = Format Date/Time String(time format string (%c)="%Y%m%d_log.txt") -> (date/time string=w930:string)  [unwired: 2 in]
                    n427 = Build Path(base path=w931, name or relative path=w930) -> (appended path=w926:path)
                    n428 = call-poly <vilib>:"Write Delimited Spreadsheet.vi"("file path (dialog if empty)"=w926, "2D data"=w927) -> ()  [unwired: 12 in, 2 out]
                    n429 = property on="Record Data" class="Bool (strict)"("DisabledEnum"=w933) -> ()  [unwired: 2 in, 2 out]
                    n430 = property on="Recording Duration [s]" class="DigNum (strict)"("DisabledEnum"=w933) -> ()  [unwired: 2 in, 2 out]
                    n431 = property on="Data Recording Progress" class="Slide (strict)"("Value"=u32 0 ("dP Recording Progress")) -> ()  [unwired: 2 in, 2 out]
                  }
                }
              }
              frame True {
                n432 = control-ref of="Data Folder"() -> (w950:refnum<vi>)
                n433 = control-ref of="Record Data"() -> (w945:refnum<vi>)
                n434 = property class="Path"(reference=w950, "DisabledEnum"=T29."Disabled and Grayed Out" ("Disabled")) -> ()  [unwired: 1 in, 2 out]
                n435 = property class="Bool (strict)"(reference=w945, "DisabledEnum"=T29."Enabled" ("Disabled")) -> ()  [unwired: 1 in, 2 out]
                n436 = control-ref of="Data Prefix"() -> (w947:refnum<vi>)
                n437 = property on="Recording Duration [s]" class="DigNum (strict)"("DisabledEnum"=T29."Disabled and Grayed Out" ("Disabled")) -> ()  [unwired: 2 in, 2 out]
                n438 = property class="Str"(reference=w947, "DisabledEnum"=T29."Disabled and Grayed Out" ("Disabled")) -> ()  [unwired: 1 in, 2 out]
                n439 = property on="Sampling\nFrequency" class="DigNum (strict)"() -> ("Value"=w941:dbl)  [unwired: 2 in, 2 out]
                n440 = property on="Recording Duration [s]" class="DigNum (strict)"() -> ("Value"=w942:dbl)  [unwired: 2 in, 2 out]
                n441 = control-ref of="Data Recording Progress"() -> (w944:refnum<vi>)
                n442 = Multiply(x=w942, y=w941) -> (x*y=w943:dbl)
                n443 = property class="Slide (strict)"(reference=w944, "Scale.Maximum"=w943) -> ()  [unwired: 1 in, 2 out]
              }
            }
          }
        }
      }
      n444 = TCP Open Connection(address=w103, remote port or service name=w104) -> (connection ID=w101:refnum<k5>, error out=w102:errorcluster)  [unwired: 1 in, 2 out]
      n445 = while {
        stop <- w688 stop-if-true
        # "Partially Reset Offset Values"
        n446 = event shown="[1] \"Zero Pressure Offsets\": Value Change" {
          selector: _ -> [_ _ _]
          dyn-events: _ -> [_ _ _]
          timeout: _ -> [_ _ _]
          tunnel: [TRUE FALSE FALSE] -> w688
          tunnel: [w689 w693 w711] -> w687
          event Timeout; "Stop": Value Change {
            n447 = event-data() -> ()  [unwired: 1 in, 3 out]
            n448 = local read "Offset Parameters"() -> (w689:T4)
          }
          event "Zero Pressure Offsets": Value Change {
            n449 = event-data() -> ("NewVal"=w692:bool)  [unwired: 1 in, 2 out]
            n450 = local read "Offset Parameters"() -> (w691:T4)
            n451 = case shown="True" w692 {
              tunnel: [w695 w700] -> w693
              tunnel: w691 -> [w695 w696]
              frame False {
              }
              frame True {
                n452 = Initialize Array(0.0 ("element"), 8 ("dimension size")) -> (w699:dbl[])
                n453 = Index Array(array=w699) -> (element #1=w701:dbl, element #2=w702:dbl, element #3=w703:dbl, element #4=w704:dbl, element #5=w705:dbl, element #6=w706:dbl, element #7=w707:dbl, element #8=w708:dbl)  [unwired: 8 in]
                n454 = Bundle By Name(cluster=w696, "Mega Tank\nPressure"=w701, "Separator Pressure"=w702, "Liquid Inlet\nPressure"=w703, "Vapor Inlet\nPressure"=w704, "Vapor Inlet\nPressure"=w705, "Test Section\nPressure"=w706, "Upper Dev Section\nPressure"=w707, "Lower Dev Section\nPressure"=w708) -> (w700:T4)
              }
            }
          }
          event "Zero Temp Offsets": Value Change {
            n455 = event-data() -> ("NewVal"=w710:bool)  [unwired: 1 in, 2 out]
            n456 = local read "Offset Parameters"() -> (w709:T4)
            n457 = case shown="True" w710 {
              tunnel: [w713 w718] -> w711
              tunnel: w709 -> [w713 w714]
              frame False {
              }
              frame True {
                n458 = Initialize Array(0.0 ("element"), 7 ("dimension size")) -> (w717:dbl[])
                n459 = Index Array(array=w717) -> (element #1=w719:dbl, element #2=w720:dbl, element #3=w721:dbl, element #4=w722:dbl, element #5=w723:dbl, element #6=w724:dbl, element #7=w725:dbl)  [unwired: 7 in]
                n460 = Bundle By Name(cluster=w714, "Mega Tank\nTemperature"=w719, "Separator \nTemperature"=w720, "Liquid Inlet\nTemperature"=w721, "Vapor Inlet\nTemperature"=w722, "Vapor Inlet \nTemperature"=w723, "Test Section\nTemperature"=w724, "Upper Dev Section\nTemperature"=w725) -> (w718:T4)
              }
            }
          }
        }
        n461 = property on="Offset Parameters" class="Clust (strict)"("Val(Sgnl)"=w687) -> ()  [unwired: 2 in, 2 out]
      }
      n462 = while {
        tunnel: w101 -> [w241]
        tunnel: [w240] -> w99
        shift-right: [w239] -> w100
        shift-left: w102 -> [w242]
        i -> [w238]
        stop <- w244 stop-if-true
        # "Liquid/vapor pump control"
        n463 = event shown="[0] Timeout" {
          selector: _ -> [_ _ _ _]
          dyn-events: _ -> [_ _ _ _]
          timeout: 100 -> [_ _ _ _]
          tunnel: [_ _ _ TRUE] -> w244
          tunnel: w242 -> [w255 w314 w346 w369]
          tunnel: w241 -> [w259 w315 w347 w370]
          tunnel: [w253 w313 w329 w358] -> w240
          tunnel: [w252 w312 w328 w357] -> w239
          tunnel: w238 -> [w258 _ _ _]
          event Timeout {
            n464 = event-data() -> ()  [unwired: 1 in, 1 out]
            n465 = case shown="1" w258 {
              tunnel: w259 -> [w281 w288]
              tunnel: [w281 w288] -> w257
              tunnel: [w280 w283] -> w256
              tunnel: w255 -> [w280 w289]
              frame 0, Default {
              }
              frame 1 {
                # "Sync PID modes"
                n466 = property on="PID Mode" class="Bool (strict)"(error in=w289) -> (error out=w287:errorcluster, "Value"=w286:bool)  [unwired: 1 in, 1 out]
                n467 = property on="PID Mode" class="Bool (strict)"(error in=w287, "Val(Sgnl)"=w286) -> (error out=w285:errorcluster)  [unwired: 1 in, 1 out]
                n468 = property on="PID Mode" class="Bool (strict)"(error in=w285) -> (error out=w284:errorcluster, "Value"=w282:bool)  [unwired: 1 in, 1 out]
                n469 = property on="PID Mode" class="Bool (strict)"(error in=w284, "Val(Sgnl)"=w282) -> (error out=w283:errorcluster)  [unwired: 1 in, 1 out]
              }
            }
            n470 = control-ref of="Flow Setpoint Adrs"() -> (w269:refnum<vi>)
            n471 = control-ref of="Pump Output Adrs"() -> (w268:refnum<vi>)
            n472 = control-ref of="Flow Setpoint Adrs"() -> (w267:refnum<vi>)
            n473 = control-ref of="Pump Output Adrs"() -> (w266:refnum<vi>)
            n474 = control-ref of="Flow Set Point [g/s]"() -> (w264:refnum<vi>)
            n475 = control-ref of="Pump Output [%]"() -> (w263:refnum<vi>)
            n476 = control-ref of="Flow Set Point [g/s]"() -> (w262:refnum<vi>)
            n477 = control-ref of="Pump Output [%]"() -> (w261:refnum<vi>)
            n478 = Build Array(w269, w268, w267, w266) -> (w265:refnum<vi>[])
            n479 = Build Array(w264, w263, w262, w261) -> (w260:refnum<vi>[])
            n480 = for {
              tunnel: w257 -> [w301]
              tunnel: w256 -> [w300]
              tunnel: [w299] -> w254
              tunnel: [w298] -> w251
              tunnel: w265 -> [w297] mode=indexing
              tunnel: w260 -> [w294] mode=indexing
              n481 = property class="DigNum (strict)"(reference=w297) -> ("Value"=w296:u16)  [unwired: 1 in, 2 out]
              n482 = call-poly <vilib>:"MB Ethernet Master Query (poly).vi"("TCP Connection Refnum in"=w301, "Starting Address"=w296, "Quantity"=u16 2, "error in"=w300) -> ("TCP Connection Refnum (dup)"=w299:refnum<k5>, "Holding Registers"=w291:u16[], "error out"=w298:errorcluster)  [unwired: 12 in, 1 out]
              n483 = Reverse 1D Array(array=w291) -> (reversed array=w290:u16[])
              n484 = Type Cast(type=sgl 0.0, x=w290) -> (*(type *) &x=w292:sgl)
              n485 = property class="DigNum (strict)"(reference=w294, "Value"=w292) -> ()  [unwired: 1 in, 2 out]
            }
            n486 = property on="Manual Mode Adrs" class="DigNum (strict)"() -> ("Value"=w249:u16)  [unwired: 2 in, 2 out]
            n487 = property on="Manual Mode Adrs" class="DigNum (strict)"() -> ("Value"=w250:u16)  [unwired: 2 in, 2 out]
            n488 = Build Array(w250, w249) -> (w248:u16[])
            n489 = control-ref of="PID Mode"() -> (w246:refnum<vi>)
            n490 = control-ref of="PID Mode"() -> (w247:refnum<vi>)
            n491 = Build Array(w247, w246) -> (w245:refnum<vi>[])
            n492 = for {
              tunnel: w254 -> [w279]
              tunnel: [w278] -> w253
              tunnel: [w277] -> w252
              tunnel: w251 -> [w276]
              tunnel: w248 -> [w275] mode=indexing
              tunnel: w245 -> [w271] mode=indexing
              n493 = call-poly <vilib>:"MB Ethernet Master Query (poly).vi"("TCP Connection Refnum in"=w279, "Starting Address"=w275, "Quantity"=u16 1, "error in"=w276) -> ("TCP Connection Refnum (dup)"=w278:refnum<k5>, "Coils"=w273:bool[], "error out"=w277:errorcluster)  [unwired: 12 in, 1 out]
              n494 = Index Array(array=w273) -> (element=w272:bool)  [unwired: 1 in]
              n495 = Not(x=w272) -> (.not. x?=w270:bool)
              n496 = property class="Bool (strict)"(reference=w271, "Value"=w270) -> ()  [unwired: 1 in, 2 out]
            }
          }
          event Value Change {
            n497 = event-data() -> ()  [unwired: 1 in, 5 out]
            n498 = control-ref of="Flow Setpoint Adrs"() -> (w311:refnum<vi>)
            n499 = control-ref of="Pump Output Adrs"() -> (w310:refnum<vi>)
            n500 = control-ref of="Flow Setpoint Adrs"() -> (w309:refnum<vi>)
            n501 = control-ref of="Pump Output Adrs"() -> (w308:refnum<vi>)
            n502 = control-ref of="Flow Set Point [g/s]"() -> (w306:refnum<vi>)
            n503 = control-ref of="Pump Output [%]"() -> (w305:refnum<vi>)
            n504 = control-ref of="Flow Set Point [g/s]"() -> (w304:refnum<vi>)
            n505 = control-ref of="Pump Output [%]"() -> (w303:refnum<vi>)
            n506 = Build Array(w311, w310, w309, w308) -> (w307:refnum<vi>[])
            n507 = Build Array(w306, w305, w304, w303) -> (w302:refnum<vi>[])
            n508 = for {
              tunnel: w315 -> [w327]
              tunnel: w314 -> [w326]
              tunnel: [w325] -> w313
              tunnel: [w324] -> w312
              tunnel: w307 -> [w323] mode=indexing
              tunnel: w302 -> [w321] mode=indexing
              n509 = property class="DigNum (strict)"(reference=w323) -> ("Value"=w322:u16)  [unwired: 1 in, 2 out]
              n510 = property class="DigNum (strict)"(reference=w321) -> ("Value"=w316:dbl)  [unwired: 1 in, 2 out]
              n511 = To Single Precision Float(number=w316) -> (single precision float=w320:sgl)
              n512 = Type Cast(type=u16[] [], x=w320) -> (*(type *) &x=w318:u16[])
              n513 = Reverse 1D Array(array=w318) -> (reversed array=w317:u16[])
              n514 = call-poly <vilib>:"MB Ethernet Master Query (poly).vi"("TCP Connection Refnum in"=w327, "Starting Address"=w322, "Registers"=w317, "error in"=w326) -> ("TCP Connection Refnum (dup)"=w325:refnum<k5>, "error out"=w324:errorcluster)  [unwired: 13 in, 1 out]
            }
          }
          event Value Change {
            n515 = event-data() -> ()  [unwired: 1 in, 3 out]
            n516 = property on="Manual Mode Request Adrs" class="DigNum (strict)"() -> ("Value"=w344:u16)  [unwired: 2 in, 2 out]
            n517 = property on="PID Mode" class="Bool (strict)"() -> ("Value"=w345:bool)  [unwired: 2 in, 2 out]
            n518 = Select(t=u16 1, s=w345, f=u16 0) -> (s? t:f=w343:u16)
            n519 = Add(x=w343, y=w344) -> (x+y=w340:u16)
            n520 = call-poly <vilib>:"MB Ethernet Master Query (poly).vi"("TCP Connection Refnum in"=w347, "Address"=w340, "Coil"=TRUE, "error in"=w346) -> ("TCP Connection Refnum (dup)"=w330:refnum<k5>, "error out"=w331:errorcluster)  [unwired: 13 in, 1 out]
            n521 = property on="Manual Mode Request Adrs" class="DigNum (strict)"() -> ("Value"=w333:u16)  [unwired: 2 in, 2 out]
            n522 = property on="PID Mode" class="Bool (strict)"() -> ("Value"=w332:bool)  [unwired: 2 in, 2 out]
            n523 = Select(t=u16 1, s=w332, f=u16 0) -> (s? t:f=w334:u16)
            n524 = Add(x=w334, y=w333) -> (x+y=w337:u16)
            n525 = call-poly <vilib>:"MB Ethernet Master Query (poly).vi"("TCP Connection Refnum in"=w330, "Address"=w337, "Coil"=TRUE, "error in"=w331) -> ("TCP Connection Refnum (dup)"=w329:refnum<k5>, "error out"=w328:errorcluster)  [unwired: 13 in, 1 out]
          }
          event "Stop": Value Change {
            n526 = event-data() -> ()  [unwired: 1 in, 3 out]
            n527 = property on="Manual Mode Request Adrs" class="DigNum (strict)"() -> ("Value"=w366:u16)  [unwired: 2 in, 2 out]
            n528 = property on="Manual Mode Request Adrs" class="DigNum (strict)"() -> ("Value"=w367:u16)  [unwired: 2 in, 2 out]
            n529 = property on="Manual Mode Adrs" class="DigNum (strict)"() -> ("Value"=w355:u16)  [unwired: 2 in, 2 out]
            n530 = property on="Manual Mode Adrs" class="DigNum (strict)"() -> ("Value"=w356:u16)  [unwired: 2 in, 2 out]
            n531 = Build Array(w367, w366) -> (w365:u16[])
            n532 = Build Array(w356, w355) -> (w354:u16[])
            n533 = control-ref of="PID Mode"() -> (w352:refnum<vi>)
            n534 = control-ref of="PID Mode"() -> (w353:refnum<vi>)
            n535 = Build Array(w353, w352) -> (w351:refnum<vi>[])
            n536 = for {
              tunnel: w370 -> [w398]
              tunnel: w369 -> [w397]
              tunnel: w365 -> [w395] mode=indexing
              tunnel: [w386] -> w362
              tunnel: [w385] -> w361
              tunnel: w354 -> [w388] mode=indexing
              tunnel: w351 -> [w387] mode=indexing
              n537 = call-poly <vilib>:"MB Ethernet Master Query (poly).vi"("TCP Connection Refnum in"=w398, "Address"=w395, "Coil"=TRUE, "error in"=w397) -> ("TCP Connection Refnum (dup)"=w390:refnum<k5>, "error out"=w389:errorcluster)  [unwired: 13 in, 1 out]
              n538 = call-poly <vilib>:"MB Ethernet Master Query (poly).vi"("TCP Connection Refnum in"=w390, "Starting Address"=w388, "Quantity"=u16 1, "error in"=w389) -> ("TCP Connection Refnum (dup)"=w386:refnum<k5>, "Coils"=w392:bool[], "error out"=w385:errorcluster)  [unwired: 12 in, 1 out]
              n539 = Index Array(array=w392) -> (element=w393:bool)  [unwired: 1 in]
              n540 = Not(x=w393) -> (.not. x?=w394:bool)
              n541 = property class="Bool (strict)"(reference=w387, "Value"=w394) -> ()  [unwired: 1 in, 2 out]
            }
            n542 = property on="Pump Output Adrs" class="DigNum (strict)"() -> ("Value"=w363:u16)  [unwired: 2 in, 2 out]
            n543 = control-ref of="Pump Output [%]"() -> (w350:refnum<vi>)
            n544 = property on="Pump Output Adrs" class="DigNum (strict)"() -> ("Value"=w364:u16)  [unwired: 2 in, 2 out]
            n545 = control-ref of="Pump Output [%]"() -> (w349:refnum<vi>)
            n546 = Build Array(w364, w363) -> (w360:u16[])
            n547 = Build Array(w350, w349) -> (w348:refnum<vi>[])
            n548 = for {
              tunnel: w362 -> [w384]
              tunnel: w361 -> [w383]
              tunnel: w360 -> [w372] mode=indexing
              tunnel: [w373] -> w358
              tunnel: [w374] -> w357
              tunnel: u16[] [0, 0] -> [w382]
              tunnel: w348 -> [w371] mode=indexing
              n549 = call-poly <vilib>:"MB Ethernet Master Query (poly).vi"("TCP Connection Refnum in"=w384, "Starting Address"=w372, "Registers"=w382, "error in"=w383) -> ("TCP Connection Refnum (dup)"=w376:refnum<k5>, "error out"=w375:errorcluster)  [unwired: 13 in, 1 out]
              n550 = call-poly <vilib>:"MB Ethernet Master Query (poly).vi"("TCP Connection Refnum in"=w376, "Starting Address"=w372, "Quantity"=u16 2, "error in"=w375) -> ("TCP Connection Refnum (dup)"=w373:refnum<k5>, "Holding Registers"=w380:u16[], "error out"=w374:errorcluster)  [unwired: 12 in, 1 out]
              n551 = Reverse 1D Array(array=w380) -> (reversed array=w381:u16[])
              n552 = Type Cast(type=sgl 0.0, x=w381) -> (*(type *) &x=w379:sgl)
              n553 = property class="DigNum (strict)"(reference=w371, "Value"=w379) -> ()  [unwired: 1 in, 2 out]
            }
          }
        }
      }
      n554 = call <vilib>:"DAQmx Stop Task.vi"("task/channels in"=w159, "error in"=w92) -> ("task out"=w174:refnum<k21>, "error out"=w175:errorcluster)  [unwired: 12 in]
      n555 = call <vilib>:"DAQmx Clear Task.vi"("task in"=w174, "error in"=w175) -> ("error out"=w176:errorcluster)  [unwired: 13 in]
      n556 = call <vilib>:"Application Directory.vi"() -> ("Application Directory"=w131:path)
      n557 = Build Path(base path=w131, name or relative path="Utility Sub VIs\\brians_diode_screen.vi") -> (appended path=w129:path)
      n558 = Open VI Reference(vi path=w129) -> (vi reference=w146:refnum<vi>, error out=w145:errorcluster)  [unwired: 5 in]
      n559 = while {
        tunnel: w146 -> [w422]
        tunnel: w145 -> [w421]
        tunnel: [w420] -> w144
        tunnel: [w419] -> w143
        stop <- w423 stop-if-true
        # "Misc. execution functions and error handling."
        n560 = event shown="[3] \"Buffer Overflow\": Value Change" {
          selector: _ -> [_ _ _ _ _]
          dyn-events: _ -> [_ _ _ _ _]
          timeout: _ -> [_ _ _ _ _]
          tunnel: [TRUE _ _ _ FALSE] -> w423
          tunnel: w422 -> [w430 _ _ _ w455]
          tunnel: w421 -> [w424 _ _ _ w454]
          tunnel: [w432 _ _ _ w453] -> w420
          tunnel: [w431 _ _ _ w452] -> w419
          event Timeout; "Stop": Value Change {
            n561 = event-data() -> ()  [unwired: 1 in, 1 out]
            n562 = property class="VI"(reference=w430, error in=w424) -> (reference out=w426:refnum<vi>, error out=w425:errorcluster, "FP.State"=w428:T34)
            n563 = Equal?(x=w428, y=T34."Closed") -> (x = y?=w429:bool)
            n564 = case shown="True" w429 {
              tunnel: [w435 w439] -> w432
              tunnel: [w434 w438] -> w431
              tunnel: w426 -> [w435 w437]
              tunnel: w425 -> [w434 w436]
              frame True {
              }
              frame False {
                n565 = invoke class="VI" method="FP.Close"(reference=w437, error in=w436) -> (reference out=w439:refnum<vi>, error out=w438:errorcluster)  [unwired: 1 in, 1 out]
              }
            }
          }
          event "Export offsets": Value Change {
            n566 = event-data() -> ("NewVal"=w440:bool)  [unwired: 1 in]
            n567 = case shown="True" w440 {
              frame False {
              }
              frame True {
                n568 = local read "Offsets"() -> (w442:T27)
                n569 = Flatten To String(anything=w442) -> (data string=w441:string)  [unwired: 3 in, 2 out]
                n570 = Write to Binary File(data=w441) -> ()  [unwired: 5 in, 3 out]
              }
            }
          }
          event "Import offsets": Value Change {
            n571 = event-data() -> ("NewVal"=w443:bool)  [unwired: 1 in, 1 out]
            n572 = case shown="True" w443 {
              frame False {
              }
              frame True {
                n573 = property on="Offsets" class="Arr (strict)"() -> ("Value"=w445:T27)  [unwired: 2 in, 2 out]
                n574 = Flatten To String(anything=w445) -> (data string=w444:string)  [unwired: 3 in, 2 out]
                n575 = Read from Binary File(5:w444) -> (0:w448:errorcluster, 2:w447:string)  [unwired: 5 in, 2 out]
                n576 = Unflatten From String(type=w445, binary string=w447, error in (no error)=w448) -> (value=w446:T27)  [unwired: 2 in, 2 out]
                n577 = property on="Offsets" class="Arr (strict)"("Val(Sgnl)"=w446) -> ()  [unwired: 2 in, 2 out]
              }
            }
          }
          event "Buffer Overflow": Value Change {
            n578 = event-data() -> ("NewVal"=w449:bool)  [unwired: 1 in]
            n579 = case shown="True" w449 {
              frame False {
              }
              frame True {
                n580 = property on="Sampling\nFrequency" class="DigNum (strict)"("Value"=100.0) -> ()  [unwired: 2 in, 2 out]
                n581 = One Button Dialog(message="The PC buffer overflowed. Check for unncessary VIs that are open and blocking main loop execution. The sampling frequency has been adjusted to 100 Hz. Adjust the rate when suspected processes has been terminated.") -> ()  [unwired: 1 in, 1 out]
              }
            }
          }
          event "Open Brians VI": Value Change {
            n582 = event-data() -> ()  [unwired: 1 in, 1 out]
            n583 = invoke class="VI" method="FP.Open"(reference=w455, error in=w454, "State"=T34."Maximized") -> (reference out=w459:refnum<vi>, error out=w458:errorcluster)  [unwired: 2 in, 3 out]
            n584 = property class="VI" props=["FP.Monitor", "FP.Monitor"](reference=w459, error in=w458, "FP.Monitor"=u16 3 ("Front Panel Window:Monitor")) -> (reference out=w453:refnum<vi>, error out=w452:errorcluster)  [unwired: 1 out]
          }
        }
      }
      n585 = control-ref of="Pump Output [%]"() -> (w76:refnum<vi>)
      n586 = control-ref of="Pump Output [%]"() -> (w75:refnum<vi>)
      n587 = control-ref of="PID Mode"() -> (w73:refnum<vi>)
      n588 = control-ref of="PID Mode"() -> (w72:refnum<vi>)
      n589 = disable-structure shown="Enabled" {
        frame Enabled {
          # "Valve Output Task"
          n590 = local read "Output"() -> (w730:T19)
          n591 = Unbundle By Name(w730) -> ("Proportional Valve Physical Channels.Vapor Valve"=w729:tag, "Proportional Valve Physical Channels.Liquid Valve"=w728:tag)
          n592 = control-ref of="Stop"() -> (w727:refnum<vi>)
          n593 = control-ref of="Valve Voltage Output"() -> (w726:refnum<vi>)
          n594 = call "valve_control_output.vi"("STOP! Refnum"=w727, "Voltage Arr Refnum"=w726, "Liquid channel"=w728, "Vapor channel"=w729) -> ()  [unwired: 2 in]
        }
        frame Disabled {
        }
      }
      n595 = Build Array(w76, w75) -> (w74:refnum<vi>[])
      n596 = Build Array(w73, w72) -> (w71:refnum<vi>[])
      n597 = while {
        tunnel: w74 -> [w182]
        tunnel: w71 -> [w181]
        tunnel: string[] ["Vapor Pump", "Liquid Pump"] -> [w180]
        stop <- w183 stop-if-true
        # "Pump max out saftey mechanism when pump reaches 100% in PID mode"
        n598 = for {
          tunnel: w182 -> [w194] mode=indexing
          tunnel: w181 -> [w188] mode=indexing
          tunnel: w180 -> [w190] mode=indexing
          tunnel: "has maxed out. Attempted to turn down to 10% in manual mode." ("string") -> [w189]
          n599 = property class="Bool (strict)"(reference=w188) -> (reference out=w184:refnum<vi>, "Value"=w186:bool)  [unwired: 1 in, 1 out]
          n600 = property class="DigNum (strict)"(reference=w194) -> (reference out=w191:refnum<vi>, "Value"=w193:dbl)  [unwired: 1 in, 1 out]
          n601 = Equal?(x=w193, y=100.0) -> (x = y?=w187:bool)
          n602 = And(x=w187, y=w186) -> (x .and. y?=w185:bool)
          n603 = case shown="True" w185 {
            tunnel: w191 -> [_ w210]
            tunnel: w184 -> [_ w208]
            tunnel: w190 -> [_ w202]
            tunnel: w189 -> [_ w195]
            frame False {
            }
            frame True {
              w204 = "msgQueue" ("name (unnamed)")
              n604 = property class="Bool (strict)"(reference=w208, "Val(Sgnl)"=FALSE ("Value (Signaling)")) -> (error out=w206:errorcluster)  [unwired: 1 in, 1 out]
              n605 = property class="DigNum (strict)"(reference=w210, error in=w206, "Val(Sgnl)"=10.0 ("Value (Signaling)")) -> (error out=w205:errorcluster)  [unwired: 1 out]
              n606 = Concatenate Strings(w202, " " ("string"), w195) -> (w199:string)
              n607 = Obtain Queue(name (unnamed)=w204, element data type=w204, create if not found? (T)=FALSE, error in (no error)=w205) -> (queue out=w201:refnum<queue>, error out=w200:errorcluster)  [unwired: 1 in, 1 out]
              n608 = Enqueue Element(queue=w201, element=w199, error in (no error)=w200) -> (queue out=w198:refnum<queue>, error out=w197:errorcluster)  [unwired: 1 in, 1 out]
              n609 = Release Queue(queue=w198, error in (no error)=w197) -> ()  [unwired: 1 in, 3 out]
            }
          }
        }
        n610 = local read "Stop"() -> (w183:bool)
        n611 = Wait (ms)(milliseconds to wait=u32 500) -> ()  [unwired: 1 out]
      }
      n612 = Close Reference(reference=w144, error in (no error)=w143) -> ()  [unwired: 1 out]
      n613 = TCP Close Connection(connection ID=w99, error in (no error)=w100) -> ()  [unwired: 1 in, 2 out]
    }
    frame #3 {
      w963 = T29."Enabled" ("Disabled")
      n614 = control-ref of="Stop"() -> (w967:refnum<vi>)
      n615 = control-ref of="System Running"() -> (w964:refnum<vi>)
      n616 = property class="Bool (strict)"(reference=w967, "Value"=FALSE) -> ()  [unwired: 1 in, 2 out]
      n617 = property class="Bool (strict)"(reference=w964, "Value"=FALSE) -> ()  [unwired: 1 in, 2 out]
      n618 = property on="Input" class="Clust (strict)"("DisabledEnum"=w963) -> ()  [unwired: 2 in, 2 out]
      n619 = property on="Safety" class="Clust (strict)"("DisabledEnum"=w963) -> ()  [unwired: 2 in, 2 out]
      n620 = property on="Commit Settings" class="Bool (strict)"("DisabledEnum"=w963) -> ()  [unwired: 2 in, 2 out]
      n621 = property on="Output" class="Clust (strict)"("DisabledEnum"=w963) -> ()  [unwired: 2 in, 2 out]
      "error out" <- w962
    }
  }
